vi "HOST_856.vi"() -> ()   [LabVIEW 2018]
uses:
  <vilib>/userdefined/High Color/nirio_resource_hc.ctl
  <instrlib>/niDCPower/nidcpower.llb/niDCPower Measurement Type.ctl
  <vilib>/FPGAPlugInAG/PXI-7953R/niLvFpga_Open_PXI-7953R.vi
  <vilib>/rvi/interface/common/dynamic/niFpgaDynamicAddResources.vi
  <vilib>/FPGAPlugInAG/Dynamic/niLvFpga_Reset_Dynamic.vi
  <vilib>/FPGAPlugInAG/Dynamic/niLvFpga_Run_Dynamic.vi
  <vilib>/Utility/error.llb/Error Cluster From Error Code.vi
  <vilib>/rvi/errors/niLvFpgaAdjustHostInterfaceError.vi
  <vilib>/FPGAPlugInAG/Dynamic/niLvFpga_Close_Dynamic.vi
  <vilib>/rvi/interface/nirviOpenFPGA/nirviOpenFPGA.xnode
  FPGA Bitfiles/856_FPGATarget_TARGET856_N743GwyKryU.lvbitx
  <vilib>/rvi/interface/nirviMethod/nirviMethod.xnode
  <vilib>/rvi/interface/nirviReadWriteControl/nirviReadWriteControl.xnode
  <vilib>/rvi/interface/nirviCloseFPGA/nirviCloseFPGA.xnode
  NiFpgaLv.dll
  <vilib>/rvi/interface/Simulation/niFpgaSimulationCallBeginRW.vi
  <vilib>/Analysis/NI_AALPro.lvlib
  <vilib>/FPGAPlugInAG/Dynamic/niLvFpga_ReadFifo_Dynamic.vi
  <vilib>/rvi/errors/niLvFpgaMergeErrorWithErrorCode.vi
panel:
  in  "Включаем автоматом?":bool
  out "2V":i32
  out "PH":i32
  out "RD":i32
  out "1V":i32
  out "-15":i32
  out "STAB":i32
  out "ADC":i32
  out "PS":i32
  out "DD":i32
  in  "НЕПРЕРЫВНО":bool
  in  "Частота?":enum16{"MIN", "MAX"}(ring)
  out "FRAME_OK":bool
  in  "Frames":path=path "C:/VPL/LabView_PRJ/DOZOR/856/FRAMES"
  in  "ПРИМЕЧАНИЕ":string
  in  "Запись Кадра":bool
  out "Image":T1(plugin-control)
  out "OUT":cluster{u16, u16, u16, u16}[][](array[cluster])
  out "FRAME":u16[][](array[numeric])
  out "Среднее":dbl
  in  "ISO":dbl=1.0
  out "СКО":dbl
  out "БД":i32
  in  "Усреднение":i32=2
  in  "Какая фотка?":string="1"
  out "Фотонная калибровка":cluster{dbl[], dbl[]}(graph)={[2945.34925, 4162.883, 5407.114, 6646.145, 7867.278, 9112.486, 10343.8485, 11629.84075, 12845.8065, 14105.4315, 15360.77375, 16587.11725, 17848.9395, 19098.027, 20350.598, 21566.6655, 22775.31325, 24040.47325, 25248.73825, 26509.4255, 27746.5745, 28973.666, 30216.06275, 31422.62225, 32653.4605, 33877.69175, 35109.20175, 36357.606, 37567.2215, 38767.47625, 39966.91875, 41163.4865, 42387.08325, 43594.03975, 44808.45875, 45970.48675, 46992.77825, 47671.652, 47865.0265, 47721.78775], [754.7077538726073, 1294.11479262345, 893.7580964968845, 980.3232389360018, 850.0287895485105, 1065.2375920249935, 1169.789721684937, 1100.165165964065, 1157.3372063515674, 1007.1309132404187, 1162.2567557572454, 1457.9632114764704, 1235.5849362859356, 1356.272022665283, 1233.965587313386, 1352.3965001901172, 1891.8062110466317, 1582.0298087255514, 1624.0064309213171, 1513.4693861032604, 1646.7886382482766, 1815.5518856486406, 2715.7512741820756, 2363.008614392699, 2216.4912798029472, 2054.855897832658, 1991.5005921076636, 2056.3553886491773, 2018.0820574154084, 2317.7418848882035, 2312.454466035146, 2381.6246235017934, 2156.6081452826106, 2313.878534130175, 2194.9621434641085, 2197.1906134834308, 3715.350346195178, 3050.689760121681, 6316.385477342978, 6689.87150748068]}
  out "Ке":dbl
  out "Светосигнальная":cluster{u8, "ДИСКРЕТ, мс":u8, dbl[]}(graph)={1, "ДИСКРЕТ, мс"=6, [2945.34925, 4162.883, 5407.114, 6646.145, 7867.278, 9112.486, 10343.8485, 11629.84075, 12845.8065, 14105.4315, 15360.77375, 16587.11725, 17848.9395, 19098.027, 20350.598, 21566.6655, 22775.31325, 24040.47325, 25248.73825, 26509.4255, 27746.5745, 28973.666, 30216.06275, 31422.62225, 32653.4605, 33877.69175, 35109.20175, 36357.606, 37567.2215, 38767.47625, 39966.91875, 41163.4865, 42387.08325, 43594.03975, 44808.45875, 45970.48675, 46992.77825, 47671.652, 47865.0265, 47721.78775]}
  out "Коэффициент наклона":dbl=207.02341506892228
  out "Ssat, АЦП":dbl
  out "Usat, В":dbl
  out "СКО выхода от выхода":cluster{dbl[], dbl[]}(graph)={[2945.34925, 4162.883, 5407.114, 6646.145, 7867.278, 9112.486, 10343.8485, 11629.84075, 12845.8065, 14105.4315, 15360.77375, 16587.11725, 17848.9395, 19098.027, 20350.598, 21566.6655, 22775.31325, 24040.47325, 25248.73825, 26509.4255, 27746.5745, 28973.666, 30216.06275, 31422.62225, 32653.4605, 33877.69175, 35109.20175, 36357.606, 37567.2215, 38767.47625, 39966.91875, 41163.4865, 42387.08325, 43594.03975, 44808.45875, 45970.48675, 46992.77825, 47671.652, 47865.0265, 47721.78775], [27.56116381795225, 39.4680052194179, 40.61277628714881, 48.477521595065056, 55.182654065838534, 67.51923353941456, 80.54674293694316, 88.70693386652474, 100.42434198938025, 112.23595038021465, 121.90756785368164, 135.55632205009846, 146.1681098589908, 159.01610695461008, 168.6889274367171, 181.34877002891415, 194.2995537044542, 205.61065872116154, 218.75093055744918, 230.2984198811404, 242.14403406030874, 255.5250241052722, 276.43391011958, 276.89883684118286, 291.2733485851393, 302.2832268581072, 315.62427374926335, 328.22661952376734, 338.672418007431, 352.34511163594993, 365.25131673273967, 377.41954602802423, 390.1457799845464, 400.77045170396485, 411.75904694827284, 399.1861749481692, 316.8742762670236, 156.11020272871326, 93.14512090147284, 141.78671742797337]}
  out "Эфф. по гор.":dbl
  out "Эфф. по верт.":dbl
  in  "ДИСКРЕТ, мс":u8=6
  in  "Кол-во итераций":i32=40
  in  "Расчет":bool
  in  "10":u8=20
  in  "PH11_1":u8=3
  in  "PH11_2":u8=13
  in  "PH21_1":u8=3
  in  "PH21_2":u8=13
  in  "RG_1":u8=3
  in  "PS4_2":u16=1371
  in  "PS4_1":u16=277
  in  "PS2_2":u16=1151
  in  "PS2_1":u16=496
  in  "2017":u16=2017
  in  "Какой канал?":enum16{"OUT1", "OUT2", "OUT3"}(ring)
  in  "文韧 世男!":bool
  in  "Линейки":bool
  in  "Сколько строк?":i32=110
  in  "Строка триггер":u16=50
  in  "PS1_2":u16=1809
  in  "PS1_1":u16=715
  in  "PS3_1":u16=934
  in  "PS3_2":u16=1589
  in  "CDS1_2":u8=13
  in  "CDS1_1":u8=5
  in  "CDS2_2":u8=16
  in  "CDS2_1":u8=2
  in  "ADC_2":u8=18
  in  "ADC_1":u8=7
  in  "RG_2":u8=5
  in  "HOR":u16=880
  in  "LOW":u8=7
  in  "HIGH":u8=18
  in  "Между кадрами, мс":u8=1
  in  "Прошить АЦП":bool
  out "АЦП прошит!":bool
  in  "Усиление (до 6)_OUT3":u8=1
  in  "Усиление (до 6)_OUT1":u8=1
  in  "Усиление (до 6)_OUT2":u8=1
  in  "Смещение, до 300_OUT1":dbl
  in  "+/- OUT1":enum16{"-", "+"}(ring)=enum."+"
  in  "Смещение, до 300_OUT3":dbl
  in  "+/- OUT3":enum16{"-", "+"}(ring)=enum."+"
  in  "Смещение, до 300_OUT2":dbl
  in  "+/- OUT2":enum16{"-", "+"}(ring)=enum."+"
  in  "2/4 V":enum16{"2V", "4V"}(ring)=enum."4V"
  in  "3CH/1CH":enum16{"3CH", "1CH"}(ring)=enum."1CH"
  out "Configuration":bool[](array[boolean])=[FALSE, FALSE, FALSE, TRUE, TRUE, FALSE, TRUE, TRUE, FALSE]
  out "ADC":bool
  out "STAB":bool
  in  "0,005":dbl=0.005 format="%#_13g"
  out "-15":bool
  out "1V":bool
  out "RD":bool
  out "PH":bool
  out "2V":bool
  out "DD":bool
  out "PS":bool
  in  "ADC, V":dbl=6.0 caption="voltage level" format="%_6p"
  in  "RD, V":dbl=14.499999999999998 caption="voltage level" format="%_6p"
  in  "PH_LOW, V":dbl=-4.000000000000002 caption="voltage level" format="%_6p"
  in  "DD, V":dbl=18.500000000000007 caption="voltage level" format="%_6p"
  in  "ADC_curlim":dbl=0.2 caption="current limit" format="%_6p"
  in  "STAB_curlim":dbl=0.2 caption="current limit" format="%_6p"
  in  "RD_curlim":dbl=0.1 caption="current limit" format="%_6p"
  in  "PH_LOW_curlim":dbl=0.1 caption="current limit" format="%_6p"
  in  "2V_curlim":dbl=0.1 caption="current limit" format="%_6p"
  in  "DD_curlim":dbl=0.1 caption="current limit" format="%_6p"
  out "ADC_cur":dbl caption="measurement" format="%_6g"
  out "STAB_cur":dbl caption="measurement" format="%_6g"
  out "RD_cur":dbl caption="measurement" format="%_6g"
  out "PH_LOW_cur":dbl caption="measurement" format="%_6g"
  out "2V_cur":dbl caption="measurement" format="%_6g"
  out "DD_cur":dbl caption="measurement" format="%_6g"
  in  "STAB, V":dbl=15.0 caption="voltage level" format="%_6p"
  in  "2V":dbl=2.0 caption="voltage level" format="%_6p"
  in  "1V":dbl=1.0 caption="voltage level" format="%_6p"
  in  "1V_curlim":dbl=0.1 caption="current limit" format="%_6p"
  out "1V_cur":dbl caption="measurement" format="%_6g"
  in  "-15_curlim":dbl=0.1 caption="current limit" format="%_6p"
  out "-15_cur":dbl caption="measurement" format="%_6g"
  in  "-15, V":dbl=-15.0 caption="voltage level" format="%_6p"
  in  "PS_LOW, V":dbl=-8.0 caption="voltage level" format="%_6p"
  in  "PS_LOW_curlim":dbl=0.1 caption="current limit" format="%_6p"
  out "PS_LOW_cur":dbl caption="measurement" format="%_6g"
  in  "Питание":bool
  in  "Стоп":bool
  in  "2":refnum<k15>="PXI1Slot4" caption="instrument handle"
  in  "0":refnum<k15>="PXI1Slot2" caption="instrument handle"
  in  "1":refnum<k15>="PXI1Slot3" caption="instrument handle"
  in  "resource name":T2="PXI1Slot5"
  in  "LOGS":path=path "C:/VPL/LabView_PRJ/DOZOR/856/LOGS"
  out "Номер образца":string="2"
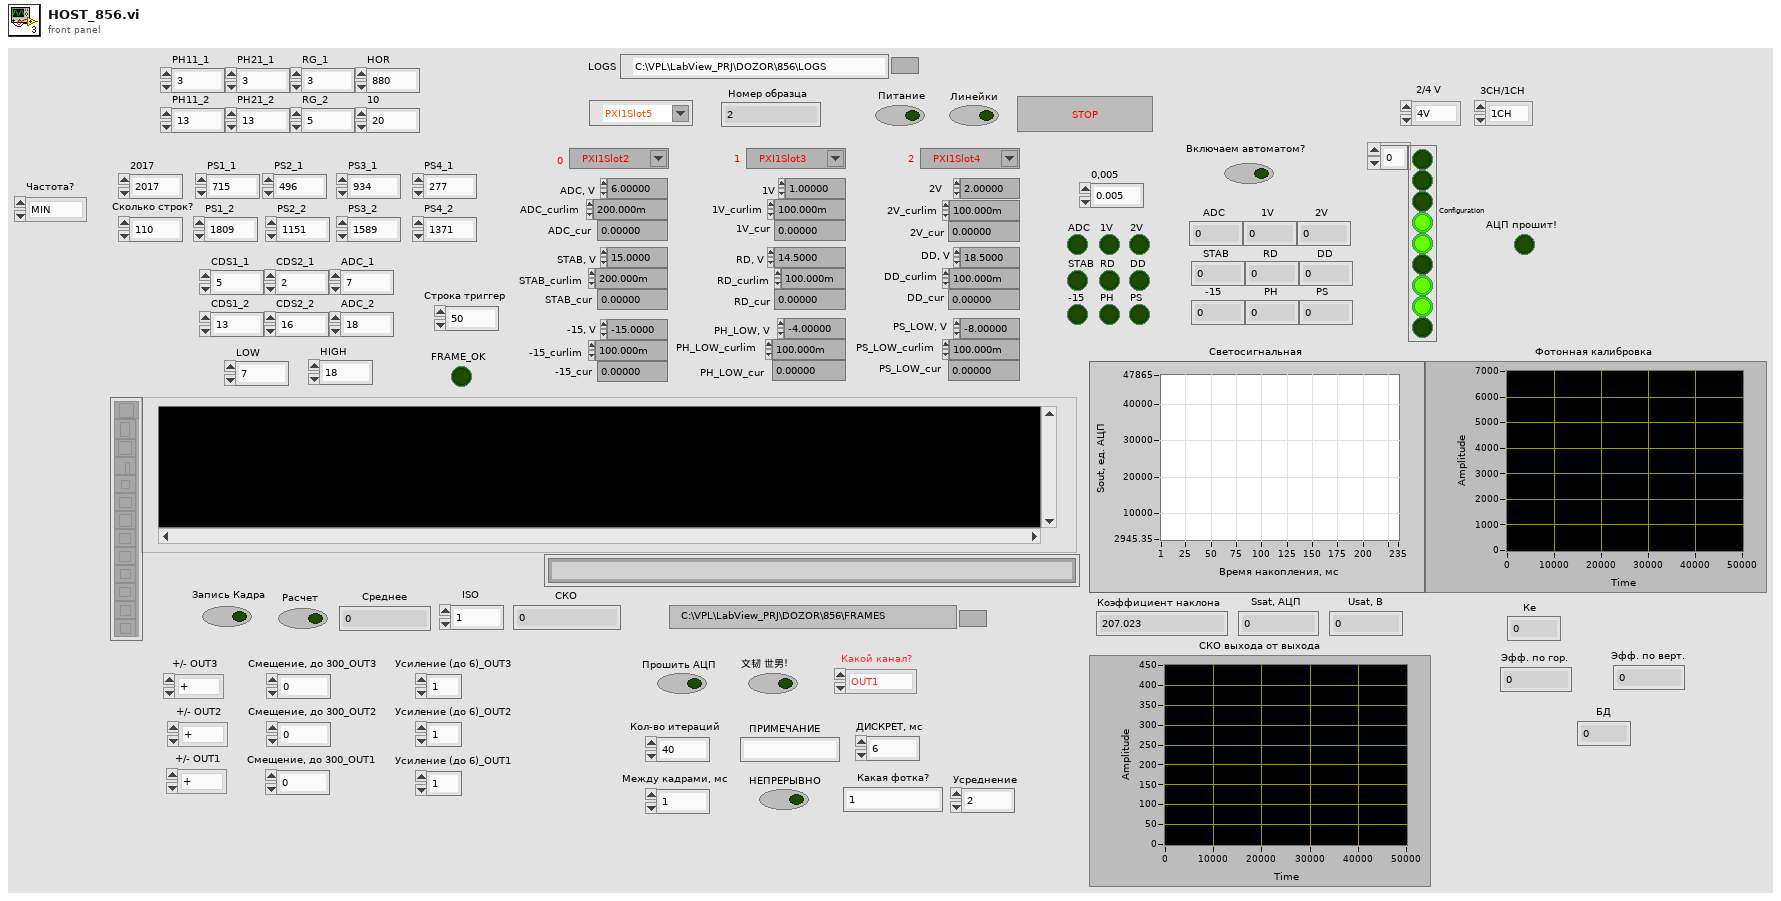
[diagram p1: front panel]
types:
  T1 = typedef "IMAQ Image.ctl" = refnum<image>
  T2 = typedef "nirio_resource_hc.ctl" = tag
  T3 = enum16{"open", "replace", "create", "open or create", "replace or create", "replace or create with confirmation"}
  T4 = typedef "niDCPower Measurement Type.ctl" = i32
  T5 = typedef "Image Type" = u32
  T6 = enum16{"Configuration", "MUX", "RED PGA", "GREEN PGA", "BLUE PGA", "RED OFF", "GREEN OFF", "BLUE OFF"}
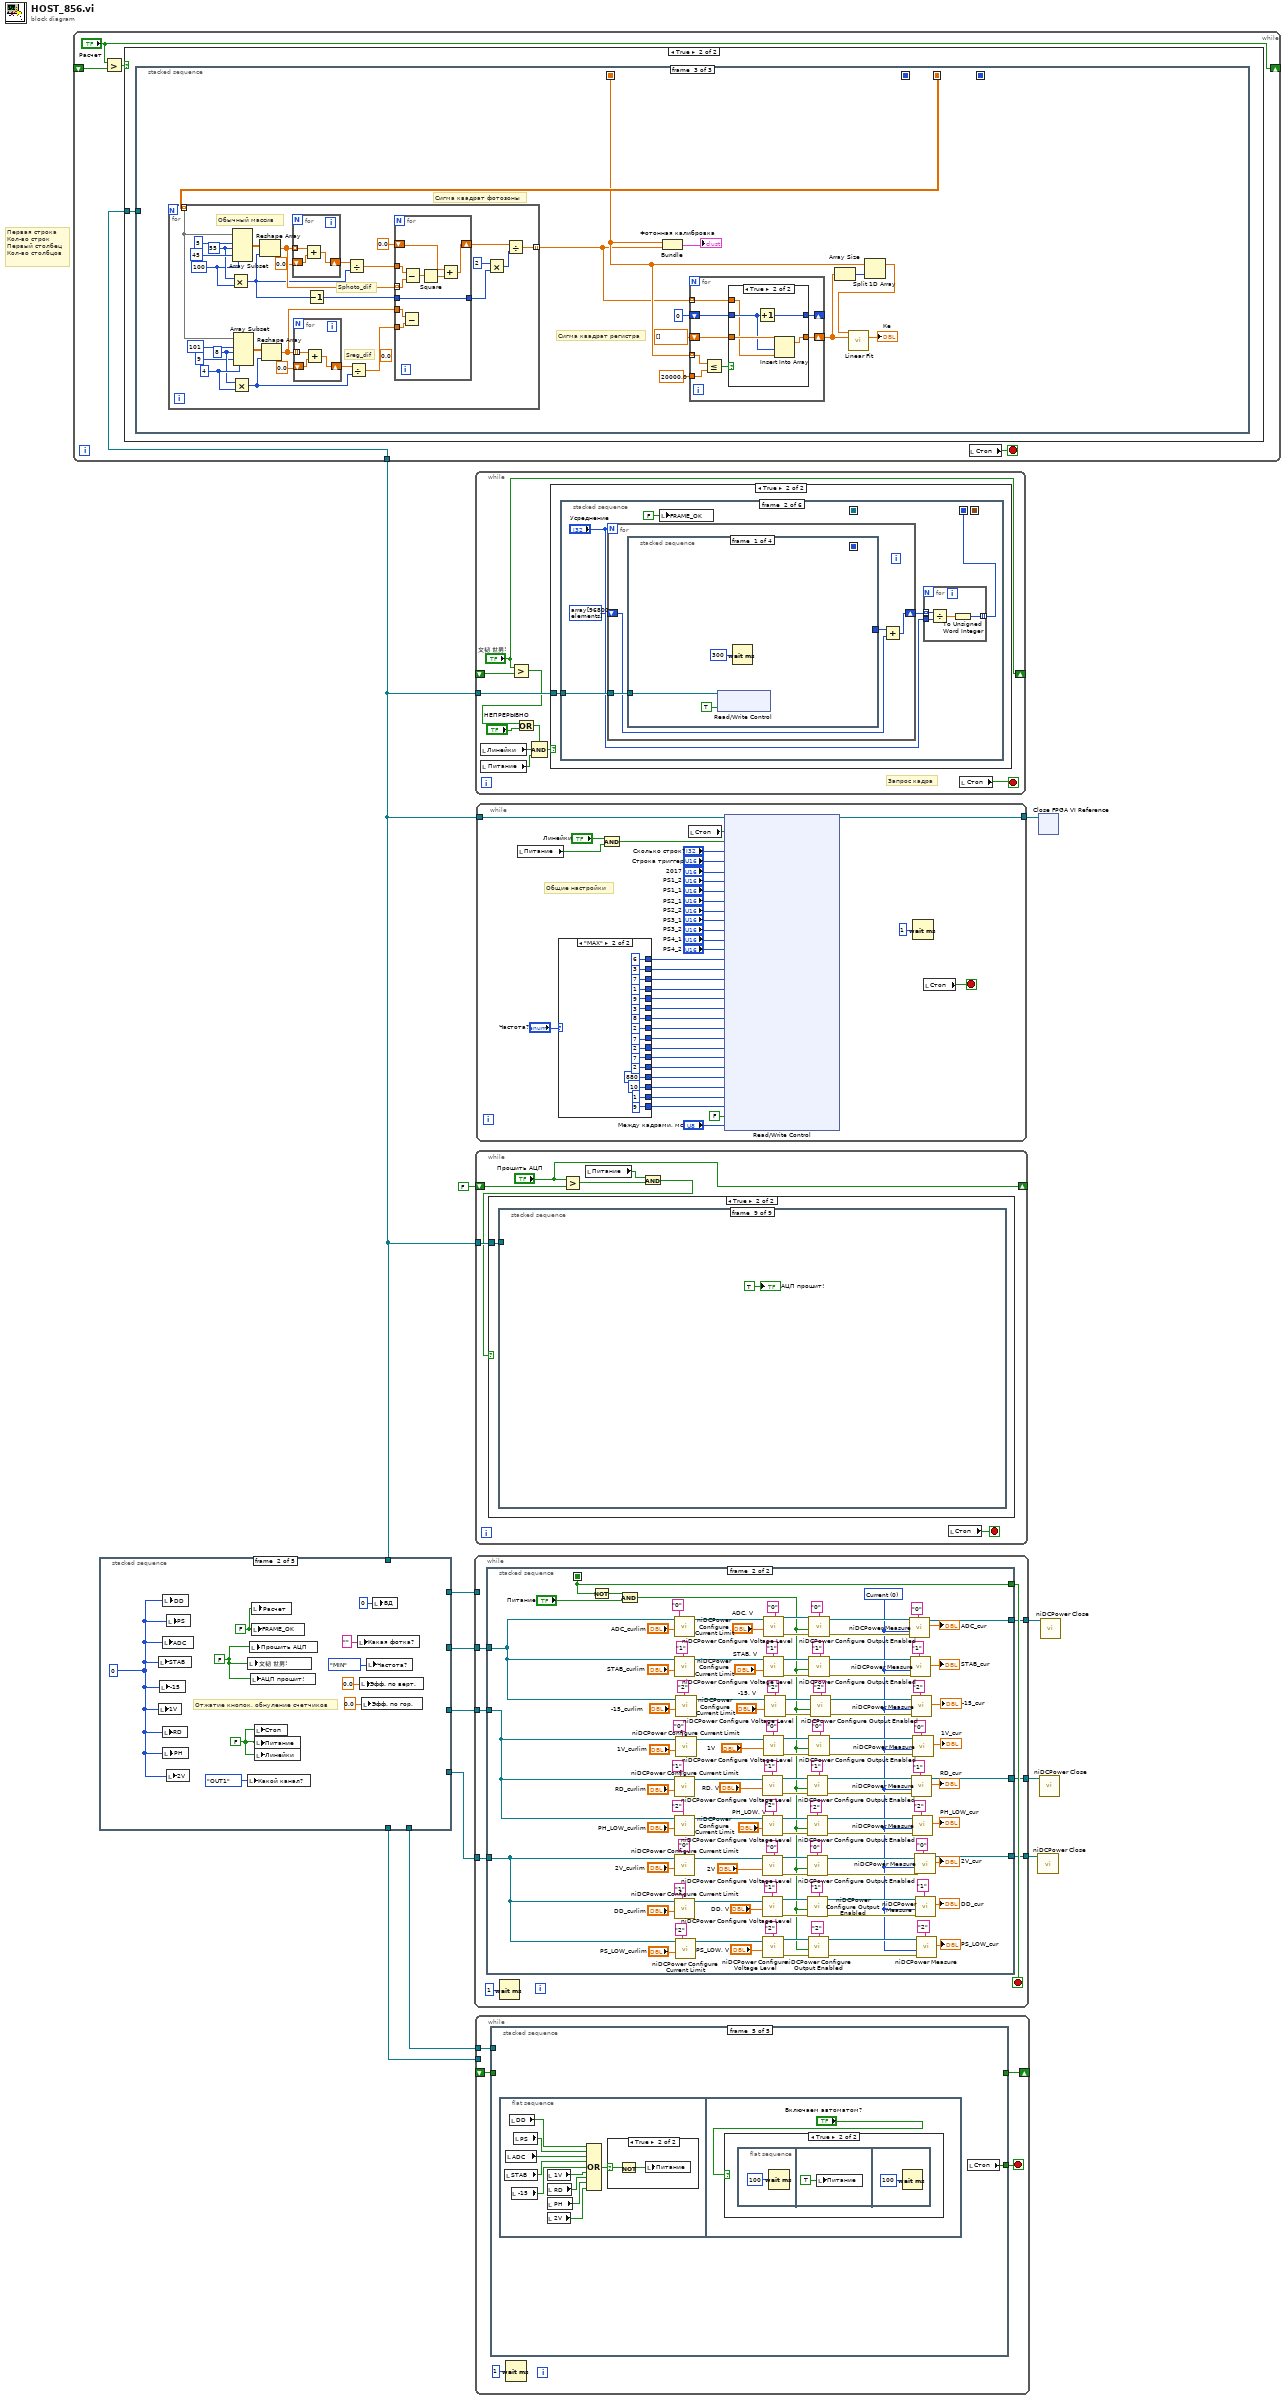
[diagram p0: block diagram]
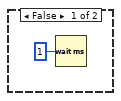
[diagram p2: hidden frame]
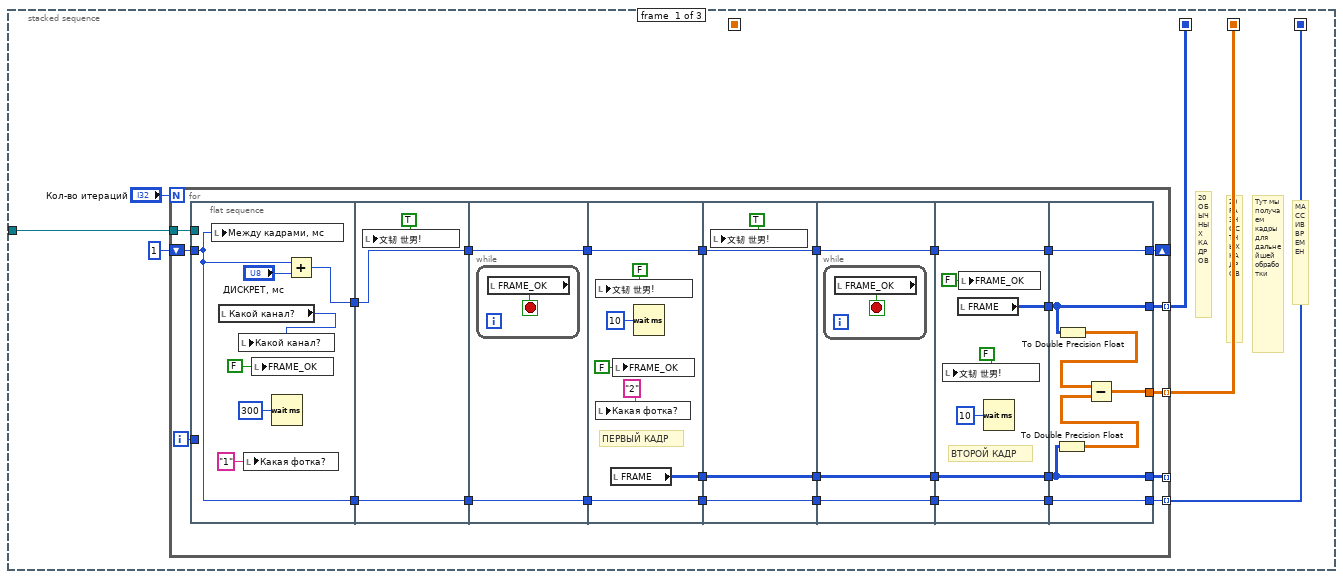
[diagram p3: hidden frame]
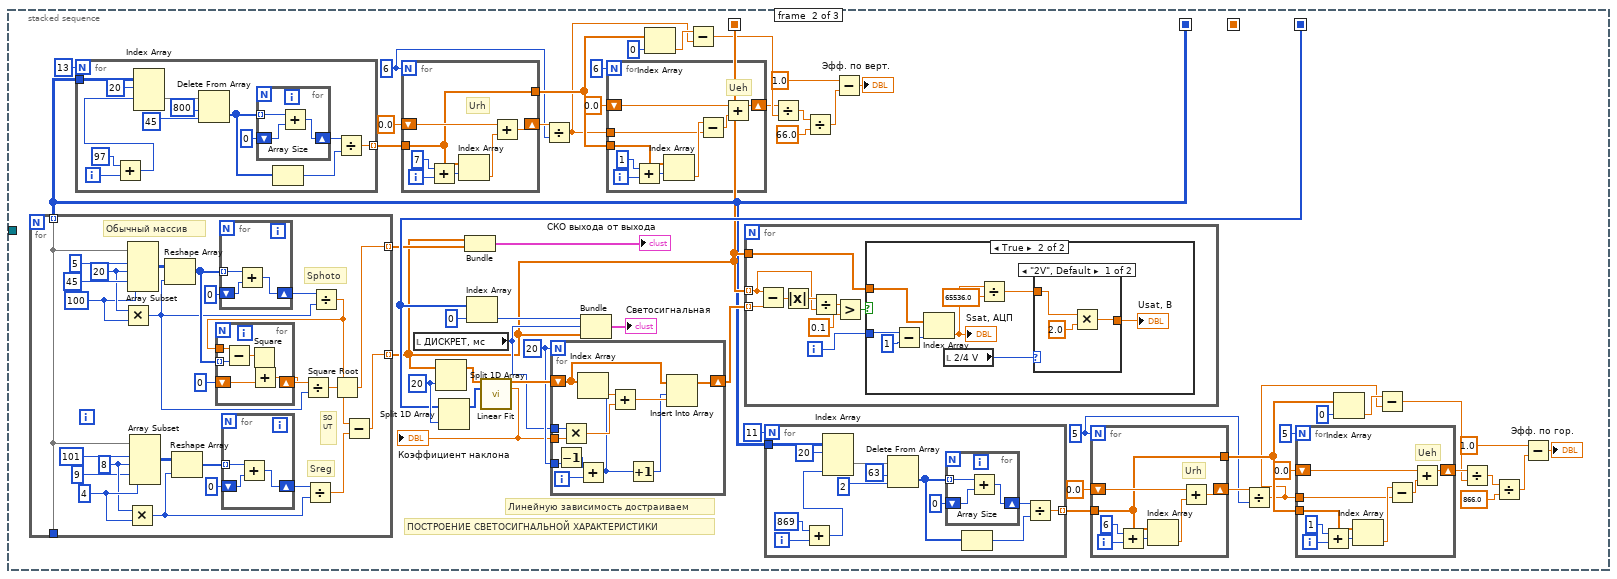
[diagram p4: hidden frame]
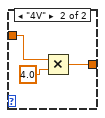
[diagram p6: hidden frame]
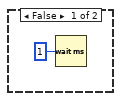
[diagram p8: hidden frame]
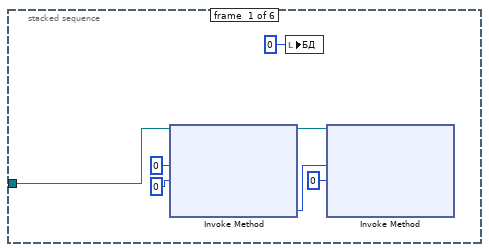
[diagram p9: hidden frame]
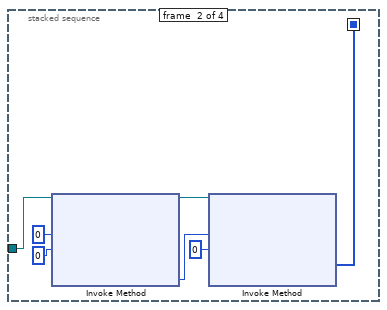
[diagram p10: hidden frame]
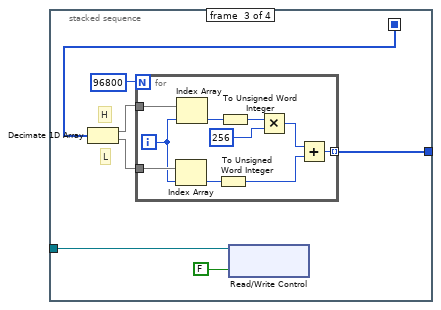
[diagram p11: hidden frame]
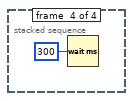
[diagram p12: hidden frame]
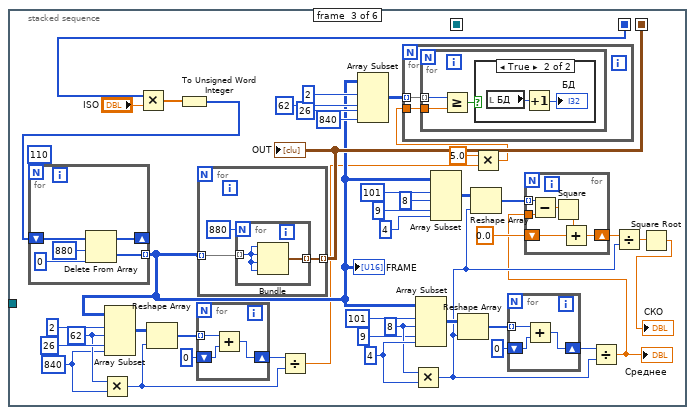
[diagram p13: hidden frame]
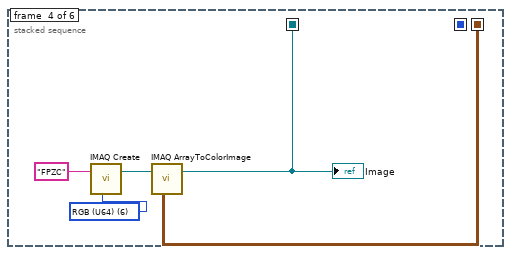
[diagram p15: hidden frame]
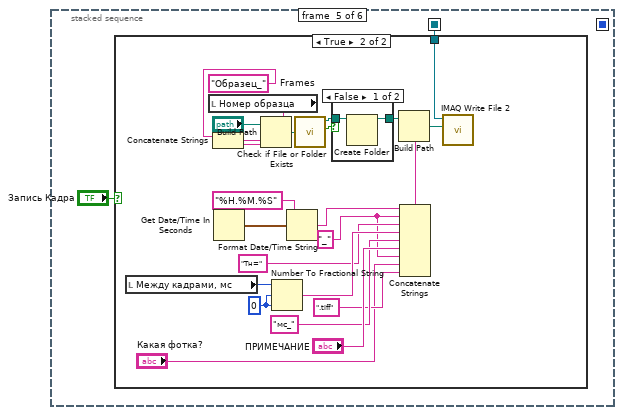
[diagram p16: hidden frame]
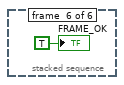
[diagram p19: hidden frame]
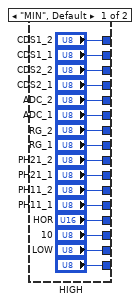
[diagram p20: hidden frame]
diagram:
  # "Первая строка\nКол-во строк\nПервый столбец\nКол-во столбцов"
  n1 = stacked-sequence {
    tunnel: [_ _ _ w61 _] -> w12
    tunnel: [_ _ _ _ w69] -> w9
    tunnel: [_ _ _ _ w68] -> w11
    tunnel: [_ _ _ _ w67] -> w10
    tunnel: [_ _ _ w61 _] -> w1
    tunnel: [_ _ _ w61 _] -> w5
    tunnel: [_ _ w24 _ _] -> w2
    frame #0 {
      n2 = call "Begin.vi"() -> ("Номер образца 2"=→"Номер образца":string)  [unwired: 11 in]
    }
    frame #1 {
      w14 = 0 ("DD")
      w21 = FALSE ("FRAME_OK")
      w22 = FALSE
      w23 = FALSE ("Стоп")
      # "Отжатие кнопок, обнуление счетчиков"
      n3 = local write "STAB"(w14) -> ()
      n4 = local write "1V"(w14) -> ()
      n5 = local write "-15"(w14) -> ()
      n6 = local write "ADC"(w14) -> ()
      n7 = local write "RD"(w14) -> ()
      n8 = local write "DD"(w14) -> ()
      n9 = local write "PH"(w14) -> ()
      n10 = local write "2V"(w14) -> ()
      n11 = local write "PS"(w14) -> ()
      n12 = local write "Какой канал?"(enum16{"OUT1", "OUT2", "OUT3"}."OUT1" ("Какой канал?")) -> ()
      n13 = local write "文韧 世男!"(w22) -> ()
      n14 = local write "Прошить АЦП"(w22) -> ()
      n15 = local write "АЦП прошит!"(w22) -> ()
      n16 = local write "FRAME_OK"(w21) -> ()
      n17 = local write "Расчет"(w21) -> ()
      n18 = local write "Стоп"(w23) -> ()
      n19 = local write "Питание"(w23) -> ()
      n20 = local write "Линейки"(w23) -> ()
      n21 = local write "Какая фотка?"("" ("Какая фотка?")) -> ()
      n22 = local write "Эфф. по верт."(0.0 ("Эфф. по верт.")) -> ()
      n23 = local write "Эфф. по гор."(0.0 ("Эфф. по гор.")) -> ()
      n24 = local write "Частота?"(enum16{"MIN", "MAX"}."MIN" ("Частота?")) -> ()
      n25 = local write "БД"(0 ("БД")) -> ()
    }
    frame #2 {
      w26 = "\t"
      n26 = local read "Номер образца"() -> (w53:string)
      n27 = Build Path(base path="LOGS", name or relative path=w53) -> (appended path=w50:path)
      n28 = Get Date/Time In Seconds() -> (seconds since 1Jan1904=w47:timestamp)
      n29 = call <vilib>:"Check if File or Folder Exists.vi"("path"=w50) -> ("file or folder exists?"=w51:bool, "dup path"=w52:path)  [unwired: 8 in, 1 out]
      n30 = Format Date/Time String(time format string (%c)="%d %H.%M.%S", seconds (now)=w47) -> (date/time string=w45:string)  [unwired: 1 in]
      n31 = case shown="False" w51 {
        tunnel: w52 -> [w59 w60]
        tunnel: [w58 w60] -> w42
        frame False {
          n32 = Create Folder(path (use dialog)=w59) -> (created path=w58:path)  [unwired: 2 in, 2 out]
        }
        frame True {
        }
      }
      n33 = Concatenate Strings(w45, ".xls" ("string")) -> (w44:string)
      n34 = Build Path(base path=w42, name or relative path=w44) -> (appended path=w46:path)
      n35 = Open/Create/Replace File(file path (use dialog)=w46, operation (0:open)=T3."open or create", access (0:read/write)=enum16{"read/write", "read-only", "write-only"}."read/write") -> (refnum out=w48:refnum<file>)  [unwired: 3 in, 2 out]
      n36 = case shown="True" TRUE {
        tunnel: w48 -> [w54 w57]
        tunnel: [w54 w55] -> w43
        frame False {
        }
        frame True {
          n37 = Set File Position(refnum=w57, from (0:start)=enum16{"start", "end", "current"}."end") -> (refnum out=w55:refnum<file>)  [unwired: 2 in, 1 out]
        }
      }
      n38 = Format Into String(initial string=w43, "Time" ("input 1"), w26, "ADC_cur", w26, "STAB_cur", w26, "-15_cur", w26, "1_cur", w26, "RD_cur", w26, "PH_LOW_cur", w26, "2V_cur", w26, "DD_cur", w26, "PS_LOW_cur", "\r\n") -> (resulting string=w24:refnum<file>)  [unwired: 2 in, 1 out]
    }
    frame #3 {
      n39 = xnode "Open FPGA VI Reference"("resource name"="resource name") -> ("FPGA VI Reference Out"=w62:refnum<k20>, "error out"=w64:errorcluster)  [unwired: 1 in]
      n40 = xnode "Invoke Method"("FPGA VI Reference In"=w62, "error in"=w64) -> ("FPGA VI Reference Out"=w65:refnum<k20>, "error out"=w63:errorcluster)
      n41 = xnode "Invoke Method"("FPGA VI Reference In"=w65, "error in"=w63) -> ("FPGA VI Reference Out"=w61:refnum<k20>)  [unwired: 1 in, 1 out]
    }
    frame #4 {
      n42 = call <instrlib>:"niDCPower Initialize.vi"("resource name"="2") -> ("error out"=w75:errorcluster, "instrument handle out"=w72:refnum<k15>)  [unwired: 3 in, 6 out]
      n43 = call <instrlib>:"niDCPower Initialize.vi"("resource name"="1") -> ("error out"=w73:errorcluster, "instrument handle out"=w70:refnum<k15>)  [unwired: 3 in, 6 out]
      n44 = call <instrlib>:"niDCPower Initialize.vi"("resource name"="0") -> ("error out"=w74:errorcluster, "instrument handle out"=w71:refnum<k15>)  [unwired: 3 in, 6 out]
      n45 = call <instrlib>:"niDCPower Configure Voltage Level.vi"("error in (no error)"=w75, "voltage level"=0.0, "channel name"="0,1,2", "instrument handle"=w72) -> ("instrument handle out"=w69:refnum<k15>)  [unwired: 6 in, 1 out]
      n46 = call <instrlib>:"niDCPower Configure Voltage Level.vi"("error in (no error)"=w73, "voltage level"=0.0, "channel name"="0,1,2", "instrument handle"=w70) -> ("instrument handle out"=w67:refnum<k15>)  [unwired: 6 in, 1 out]
      n47 = call <instrlib>:"niDCPower Configure Voltage Level.vi"("error in (no error)"=w74, "voltage level"=0.0, "channel name"="0,1,2", "instrument handle"=w71) -> ("instrument handle out"=w68:refnum<k15>)  [unwired: 6 in, 1 out]
    }
  }
  n48 = while {
    shift-right: ["Расчет"] -> _
    shift-left: _ -> [w87]
    tunnel: w1 -> [w85]
    stop <- w89 stop-if-true
    n49 = Greater?(x="Расчет", y=w87) -> (0:w88:bool)
    n50 = case shown="True" w88 {
      tunnel: w85 -> [_ w91]
      frame False {
        n51 = Wait (ms)(milliseconds to wait=u32 1) -> ()  [unwired: 1 out]
      }
      frame True {
        n52 = stacked-sequence {
          seq-local: [w92 _ _] -> [_ w167 _]
          seq-local: [w94 _ _] -> [_ _ w367]
          seq-local: [w93 _ _] -> [_ w209 _]
          seq-local: [_ w204 _] -> [_ _ w359]
          tunnel: w91 -> [w97 _ _]
          frame #0 {
            # "МАССИВ ВРЕМЕН"
            # "Тут мы получаем кадры\nдля дальнейшей обработки"
            # "20 РАЗНОСТНЫХ КАДРОВ"
            # "20 ОБЫЧНЫХ КАДРОВ"
            n53 = for {
              N: "Кол-во итераций" -> [_]
              tunnel: w97 -> [w124]
              shift-right: [w122] -> _
              shift-left: u8 1 -> [w123]
              tunnel: [w109] -> w92 mode=indexing
              tunnel: [w108] -> w94 mode=indexing
              tunnel: [w107] -> w93 mode=indexing
              tunnel: [w98] -> _ mode=indexing
              i -> [w99]
              n54 = flat-sequence {
                tunnel: w124 -> [_]
                tunnel: w123 -> [w127]
                tunnel: [w130] -> w119
                tunnel: [w127] -> w100
                tunnel: w99 -> [_]
                tunnel: [w134] -> w121
                tunnel: w119 -> [w134]
                tunnel: [w132] -> w101
                tunnel: w100 -> [w132]
                tunnel: w121 -> [w136]
                tunnel: [w136] -> w120
                tunnel: [w135] -> w102
                tunnel: w101 -> [w135]
                tunnel: w120 -> [w144]
                tunnel: [w144] -> w118
                tunnel: [w141] -> w110
                tunnel: [w139] -> w103
                tunnel: w102 -> [w139]
                tunnel: w118 -> [w148]
                tunnel: [w148] -> w117
                tunnel: [w146] -> w111
                tunnel: w110 -> [w146]
                tunnel: [w145] -> w104
                tunnel: w103 -> [w145]
                tunnel: w117 -> [w151]
                tunnel: [w151] -> w116
                tunnel: [w150] -> w112
                tunnel: w111 -> [w150]
                tunnel: [w149] -> w105
                tunnel: w104 -> [w149]
                tunnel: w116 -> [w159]
                tunnel: [w159] -> w115
                tunnel: [w158] -> w114
                tunnel: [w157] -> w113
                tunnel: w112 -> [w157]
                tunnel: [w153] -> w106
                tunnel: w105 -> [w153]
                tunnel: [w166] -> w122
                tunnel: w115 -> [w166]
                tunnel: w114 -> [w164]
                tunnel: w113 -> [w160]
                tunnel: [w163] -> w108
                tunnel: [w164] -> w109
                tunnel: [w165] -> w107
                tunnel: w106 -> [w165]
                tunnel: [w160] -> w98
                frame #0 {
                  n55 = local write "Между кадрами, мс"(w127) -> ()
                  n56 = local read "Какой канал?"() -> (w126:enum16{"OUT1", "OUT2", "OUT3"})
                  n57 = local write "Какой канал?"(w126) -> ()
                  n58 = local write "Какая фотка?"("1" ("Какая фотка?")) -> ()
                  n59 = local write "FRAME_OK"(FALSE ("FRAME_OK")) -> ()
                  n60 = Wait (ms)(milliseconds to wait=u32 300) -> ()  [unwired: 1 out]
                  n61 = Add(x=w127, y="ДИСКРЕТ, мс") -> (x+y=w130:u8)
                }
                frame #1 {
                  n62 = local write "文韧 世男!"(TRUE ("文韧 世男!")) -> ()
                }
                frame #2 {
                  n63 = while {
                    stop <- w137 stop-if-true
                    n64 = local read "FRAME_OK"() -> (w137:bool)
                  }
                }
                frame #3 {
                  # "ПЕРВЫЙ КАДР"
                  n65 = local write "文韧 世男!"(FALSE ("文韧 世男!")) -> ()
                  n66 = local write "Какая фотка?"("2" ("Какая фотка?")) -> ()
                  n67 = local read "FRAME"() -> (w141:u16[][])
                  n68 = local write "FRAME_OK"(FALSE ("FRAME_OK")) -> ()
                  n69 = Wait (ms)(milliseconds to wait=u32 10) -> ()  [unwired: 1 out]
                }
                frame #4 {
                  n70 = local write "文韧 世男!"(TRUE ("文韧 世男!")) -> ()
                }
                frame #5 {
                  n71 = while {
                    stop <- w152 stop-if-true
                    n72 = local read "FRAME_OK"() -> (w152:bool)
                  }
                }
                frame #6 {
                  # "ВТОРОЙ КАДР"
                  n73 = local write "文韧 世男!"(FALSE ("文韧 世男!")) -> ()
                  n74 = local read "FRAME"() -> (w158:u16[][])
                  n75 = local write "FRAME_OK"(FALSE ("FRAME_OK")) -> ()
                  n76 = Wait (ms)(milliseconds to wait=u32 10) -> ()  [unwired: 1 out]
                }
                frame #7 {
                  n77 = To Double Precision Float(number=w160) -> (double precision float=w161:dbl[][])
                  n78 = To Double Precision Float(number=w164) -> (double precision float=w162:dbl[][])
                  n79 = Subtract(x=w162, y=w161) -> (x-y=w163:dbl[][])
                }
              }
            }
          }
          frame #1 {
            w169 = 6
            w170 = 5
            w212 = 20
            w217 = 20 ("index")
            # "ПОСТРОЕНИЕ СВЕТОСИГНАЛЬНОЙ ХАРАКТЕРИСТИКИ"
            # "Линейную зависимость достраиваем"
            n80 = for {
              tunnel: w167 -> [w319] mode=indexing
              tunnel: [w321] -> w204 mode=indexing
              tunnel: [w325] -> w206 mode=indexing
              tunnel: [w319] -> _
              w332 = 4 ("length")
              w331 = 8 ("length")
              w341 = 100 ("length")
              w342 = 20 ("length")
              # "SOUT"
              # "Sreg"
              # "Sphoto"
              # "Обычный массив"
              n81 = Multiply(x=w342, y=w341) -> (x*y=w323:i32)
              n82 = Multiply(x=w331, y=w332) -> (x*y=w337:i32)
              n83 = Array Subset(array=w319, index (row)=5 ("index"), length (row)=w342, index (col)=45 ("index"), length (col)=w341) -> (w340:u16[][])
              n84 = Array Subset(array=w319, index (row)=101 ("index"), length (row)=w331, index (col)=9 ("index"), length (col)=w332) -> (w333:u16[][])
              n85 = Reshape Array(w340, w323) -> (w327:u16[])
              n86 = Reshape Array(w333, w337) -> (w334:u16[])
              n87 = for {
                tunnel: w327 -> [w356] mode=indexing
                shift-right: [w354] -> w338
                shift-left: u64 0 -> [w355]
                n88 = Add(x=w356, y=w355) -> (x+y=w354:u64)
              }
              n89 = for {
                tunnel: w334 -> [w353] mode=indexing
                shift-right: [w351] -> w336
                shift-left: u64 0 -> [w352]
                n90 = Add(x=w353, y=w352) -> (x+y=w351:u64)
              }
              n91 = Divide(x=w336, y=w337) -> (x/y=w328:dbl)
              n92 = Divide(x=w338, y=w323) -> (x/y=w320:dbl)
              n93 = for {
                tunnel: w327 -> [w350] mode=indexing
                shift-right: [w349] -> w324
                shift-left: u64 0 -> [w346]
                tunnel: w320 -> [w345]
                n94 = Subtract(x=w345, y=w350) -> (x-y=w348:dbl)
                n95 = Square(x=w348) -> (x^2=w347:dbl)
                n96 = Add(x=w347, y=w346) -> (x+y=w349:dbl)
              }
              n97 = Divide(x=w324, y=w323) -> (x/y=w322:dbl)
              n98 = Square Root(x=w322) -> (sqrt(x)=w325:dbl)
              n99 = Subtract(x=w320, y=w328) -> (x-y=w321:dbl)
            }
            n100 = for {
              N: 13 -> [_]
              tunnel: w167 -> [w247]
              tunnel: [w236] -> w176 mode=indexing
              i -> [w238]
              n101 = Add(x=97, y=w238) -> (x+y=w235:i32)
              n102 = Index Array(array=w247, index (dim 0)=20 ("disabled index (page)"), index (dim 1)=w235) -> (element=w245:u16[])  [unwired: 1 in]
              n103 = Delete From Array(array=w245, length=800, index=45) -> (deleted portion=w240:u16[])  [unwired: 1 out]
              n104 = for {
                tunnel: w240 -> [w250] mode=indexing
                shift-right: [w248] -> w241
                shift-left: 0 -> [w249]
                n105 = Add(x=w250, y=w249) -> (x+y=w248:i32)
              }
              n106 = Array Size(array=w240) -> (size(s)=w239:i32)
              n107 = Divide(x=w241, y=w239) -> (x/y=w236:dbl)
            }
            n108 = for {
              N: w169 -> [_]
              tunnel: w176 -> [w228]
              shift-right: [w229] -> w172
              shift-left: 0.0 -> [w231]
              tunnel: [w228] -> w181
              i -> [w234]
              # "Urh"
              n109 = Add(x=7, y=w234) -> (x+y=w232:i32)
              n110 = Index Array(array=w228, index=w232) -> (element=w230:dbl)
              n111 = Add(x=w231, y=w230) -> (x+y=w229:dbl)
            }
            n112 = local read "ДИСКРЕТ, мс"() -> (w210:u8)
            n113 = Split 1D Array(array=w204, index=w217) -> (first subarray=w216:dbl[])  [unwired: 1 out]
            n114 = Split 1D Array(array=w209, index=w217) -> (first subarray=w215:u8[])  [unwired: 1 out]
            n115 = Bundle(w204, w206) -> (→"СКО выхода от выхода":cluster{dbl[], dbl[]})  [unwired: 1 in]
            n116 = Index Array(array=w209, index=0) -> (element=w214:u8)
            n117 = call <vilib>:"Linear Fit.vi"("Y"=w216, "X"=w215) -> ("Best Linear Fit"=w213:dbl[], "slope"=w211:dbl)  [unwired: 9 in, 3 out]
            "Коэффициент наклона" <- w211
            n118 = Divide(x=w172, y=w169) -> (x/y=w168:dbl)
            n119 = for {
              N: w212 -> [_]
              tunnel: w212 -> [w308]
              shift-right: [w316] -> w208
              shift-left: w213 -> [w309]
              tunnel: w211 -> [w315]
              tunnel: w210 -> [w314]
              i -> [w318]
              n120 = Decrement(x=w308) -> (x-1=w307:i32)
              n121 = Multiply(x=w314, y=w315) -> (x*y=w313:dbl)
              n122 = Add(x=w307, y=w318) -> (x+y=w311:i32)
              n123 = Index Array(array=w309, index=w311) -> (element=w317:dbl)
              n124 = Add(x=w317, y=w313) -> (x+y=w312:dbl)
              n125 = Increment(x=w311) -> (x+1=w310:i32)
              n126 = Insert Into Array(array=w309, index=w310, new element=w312) -> (w316:dbl[])
            }
            n127 = Bundle(w214, "ДИСКРЕТ, мс"=w210, w204) -> (→"Светосигнальная":cluster{u8, "ДИСКРЕТ, мс":u8, dbl[]})  [unwired: 1 in]
            n128 = for {
              N: 6 -> [_]
              tunnel: w181 -> [w224]
              shift-right: [w219] -> w179
              shift-left: 0.0 -> [w220]
              tunnel: w168 -> [w222]
              i -> [w227]
              # "Ueh"
              n129 = Add(x=1, y=w227) -> (x+y=w225:i32)
              n130 = Index Array(array=w224, index=w225) -> (element=w223:dbl)
              n131 = Subtract(x=w223, y=w222) -> (x-y=w221:dbl)
              n132 = Add(x=w220, y=w221) -> (x+y=w219:dbl)
            }
            n133 = Index Array(array=w181, index=0) -> (element=w182:dbl)
            n134 = Subtract(x=w182, y=w168) -> (x-y=w183:dbl)
            n135 = for {
              tunnel: w204 -> [w283] mode=indexing
              tunnel: w208 -> [w291] mode=indexing
              tunnel: w204 -> [w286]
              i -> [w287]
              n136 = Subtract(x=w283, y=w291) -> (x-y=w284:dbl)
              n137 = Absolute Value(x=w284) -> (abs(x)=w285:dbl)
              n138 = Divide(x=w285, y=w283) -> (x/y=w290:dbl)
              n139 = Greater?(x=w290, y=0.1) -> (0:w288:bool)
              n140 = case shown="True" w288 {
                tunnel: w287 -> [_ w294]
                tunnel: w286 -> [_ w300]
                frame False {
                }
                frame True {
                  n141 = Subtract(x=w294, y=1) -> (x-y=w295:i32)
                  n142 = Index Array(array=w300, index=w295) -> (element=w298:dbl)
                  "Ssat, АЦП" <- w298
                  n143 = local read "2/4 V"() -> (w299:enum16{"2V", "4V"})
                  n144 = Divide(x=w298, y=65536.0) -> (x/y=w296:dbl)
                  n145 = case shown="\"2V\", Default" w299 {
                    tunnel: w296 -> [w302 w306]
                    tunnel: [w301 w304] -> w292
                    frame "2V", Default {
                      n146 = Multiply(x=w302, y=2.0) -> (x*y=w301:dbl)
                    }
                    frame "4V" {
                      n147 = Multiply(x=w306, y=4.0) -> (x*y=w304:dbl)
                    }
                  }
                  "Usat, В" <- w292
                }
              }
            }
            n148 = for {
              N: 11 -> [_]
              tunnel: w167 -> [w279]
              tunnel: [w267] -> w202 mode=indexing
              i -> [w270]
              n149 = Add(x=869, y=w270) -> (x+y=w268:i32)
              n150 = Index Array(array=w279, index (dim 0)=20 ("disabled index (page)"), index (dim 2)=w268) -> (element=w277:u16[])  [unwired: 1 in]
              n151 = Delete From Array(array=w277, length=63, index=2) -> (deleted portion=w272:u16[])  [unwired: 1 out]
              n152 = for {
                tunnel: w272 -> [w282] mode=indexing
                shift-right: [w280] -> w273
                shift-left: 0 -> [w281]
                n153 = Add(x=w282, y=w281) -> (x+y=w280:i32)
              }
              n154 = Array Size(array=w272) -> (size(s)=w271:i32)
              n155 = Divide(x=w273, y=w271) -> (x/y=w267:dbl)
            }
            n156 = Divide(x=w179, y=w183) -> (x/y=w185:dbl)
            n157 = Divide(x=w185, y=66.0) -> (x/y=w187:dbl)
            n158 = Subtract(x=1.0, y=w187) -> (x-y=→"Эфф. по верт.":dbl)
            n159 = for {
              N: w170 -> [_]
              tunnel: w202 -> [w260]
              shift-right: [w261] -> w195
              shift-left: 0.0 -> [w263]
              tunnel: [w260] -> w197
              i -> [w266]
              # "Urh"
              n160 = Add(x=6, y=w266) -> (x+y=w264:i32)
              n161 = Index Array(array=w260, index=w264) -> (element=w262:dbl)
              n162 = Add(x=w263, y=w262) -> (x+y=w261:dbl)
            }
            n163 = Divide(x=w195, y=w170) -> (x/y=w171:dbl)
            n164 = for {
              N: 5 -> [_]
              tunnel: w197 -> [w256]
              shift-right: [w251] -> w199
              shift-left: 0.0 -> [w252]
              tunnel: w171 -> [w254]
              i -> [w259]
              # "Ueh"
              n165 = Add(x=1, y=w259) -> (x+y=w257:i32)
              n166 = Index Array(array=w256, index=w257) -> (element=w255:dbl)
              n167 = Subtract(x=w255, y=w254) -> (x-y=w253:dbl)
              n168 = Add(x=w252, y=w253) -> (x+y=w251:dbl)
            }
            n169 = Index Array(array=w197, index=0) -> (element=w196:dbl)
            n170 = Subtract(x=w196, y=w171) -> (x-y=w194:dbl)
            n171 = Divide(x=w199, y=w194) -> (x/y=w192:dbl)
            n172 = Divide(x=w192, y=866.0) -> (x/y=w190:dbl)
            n173 = Subtract(x=1.0, y=w190) -> (x-y=→"Эфф. по гор.":dbl)
          }
          frame #2 {
            # "Сигма квадрат регистра"
            # "Сигма квадрат фотозоны"
            n174 = for {
              tunnel: w367 -> [w398] mode=indexing
              tunnel: [w383] -> w358 mode=indexing
              (unwired) 0.0
              w402 = 4 ("length")
              w401 = 8 ("length")
              w407 = 100 ("length")
              w408 = 55 ("length")
              # "Sreg_dif"
              # "Sphoto_dif"
              # "Обычный массив"
              n175 = Multiply(x=w408, y=w407) -> (x*y=w393:i32)
              n176 = Multiply(x=w401, y=w402) -> (x*y=w391:i32)
              n177 = Array Subset(array=w398, index (row)=5 ("index"), length (row)=w408, index (col)=45 ("index"), length (col)=w407) -> (w406:dbl[][])
              n178 = Array Subset(array=w398, index (row)=101 ("index"), length (row)=w401, index (col)=9 ("index"), length (col)=w402) -> (w403:dbl[][])
              n179 = Reshape Array(w406, w393) -> (w396:dbl[])
              n180 = Reshape Array(w403, w391) -> (w395:dbl[])
              n181 = for {
                tunnel: w396 -> [w425] mode=indexing
                shift-right: [w423] -> w405
                shift-left: 0.0 -> [w424]
                n182 = Add(x=w425, y=w424) -> (x+y=w423:dbl)
              }
              n183 = for {
                tunnel: w395 -> [w422] mode=indexing
                shift-right: [w420] -> w404
                shift-left: 0.0 -> [w421]
                n184 = Add(x=w422, y=w421) -> (x+y=w420:dbl)
              }
              n185 = Decrement(x=w393) -> (x-1=w392:i32)
              n186 = Divide(x=w405, y=w393) -> (x/y=w387:dbl)
              n187 = Divide(x=w404, y=w391) -> (x/y=w397:dbl)
              n188 = for {
                tunnel: w387 -> [w417]
                tunnel: w397 -> [w418]
                tunnel: w396 -> [w416] mode=indexing
                tunnel: w395 -> [w419]
                shift-right: [w412] -> w394
                shift-left: 0.0 -> [w413]
                tunnel: [w411] -> w388
                tunnel: w392 -> [w411]
                n189 = Subtract(x=w419, y=w418) -> ()  [unwired: 1 out]
                n190 = Subtract(x=w417, y=w416) -> (x-y=w415:dbl)
                n191 = Square(x=w415) -> (x^2=w414:dbl)
                n192 = Add(x=w413, y=w414) -> (x+y=w412:dbl)
              }
              n193 = Multiply(x=2, y=w388) -> (x*y=w389:i32)
              n194 = Divide(x=w394, y=w389) -> (x/y=w383:dbl)
            }
            n195 = Bundle(w359, w358) -> (→"Фотонная калибровка":cluster{dbl[], dbl[]})  [unwired: 1 in]
            n196 = for {
              tunnel: w359 -> [w373] mode=indexing
              tunnel: 20000.0 -> [w375]
              shift-right: [w369] -> w364
              shift-left: dbl[] [] -> [w372]
              shift-right: [w370] -> _
              shift-left: 0 -> [w371]
              tunnel: w358 -> [w368] mode=indexing
              n197 = Less Or Equal?(x=w373, y=w375) -> (x <= y?=w374:bool)
              n198 = case shown="True" w374 {
                tunnel: w372 -> [w376 w382]
                tunnel: w371 -> [w377 w380]
                tunnel: [w377 w381] -> w370
                tunnel: [w376 w379] -> w369
                tunnel: w368 -> [_ w378]
                frame False {
                }
                frame True {
                  n199 = Increment(x=w380) -> (x+1=w381:i32)
                  n200 = Insert Into Array(array=w382, index=w380, new element=w378) -> (w379:dbl[])
                }
              }
            }
            n201 = Array Size(array=w364) -> (size(s)=w363:i32)
            n202 = Split 1D Array(array=w359, index=w363) -> (first subarray=w362:dbl[])  [unwired: 1 out]
            n203 = call <vilib>:"Linear Fit.vi"("Y"=w362, "X"=w364) -> ("slope"=→"Ке":dbl)  [unwired: 9 in, 4 out]
          }
        }
      }
    }
    n204 = local read "Стоп"() -> (w89:bool)
  }
  n205 = while {
    tunnel: w12 -> [_]
    tunnel: w11 -> [w432]
    tunnel: w10 -> [w431]
    tunnel: w9 -> [w430]
    tunnel: [w428] -> w8
    tunnel: [w427] -> w7
    tunnel: [w426] -> w6
    stop <- w429 stop-if-true
    n206 = stacked-sequence {
      seq-local: ["Стоп" _] -> [_ w435]
      tunnel: w430 -> [_ w440]
      tunnel: [_ w481] -> w428
      tunnel: [_ w480] -> w427
      tunnel: [_ w479] -> w426
      tunnel: w432 -> [_ w439]
      tunnel: w431 -> [_ w438]
      tunnel: [_ w435] -> w429
      frame #0 {
      }
      frame #1 {
        w441 = T4 0 items=["Current", "Voltage"] ("measurement type")
        n207 = Not(x=w435) -> (.not. x?=w454:bool)
        n208 = And(x=w454, y="Питание") -> (x .and. y?=w436:bool)
        n209 = call <instrlib>:"niDCPower Configure Current Limit.vi"("current limit"="ADC_curlim", "channel name"="0", "instrument handle"=w439) -> ("instrument handle out"=w516:refnum<k15>)  [unwired: 7 in, 1 out]
        n210 = call <instrlib>:"niDCPower Configure Current Limit.vi"("current limit"="STAB_curlim", "channel name"="1", "instrument handle"=w439) -> ("instrument handle out"=w517:refnum<k15>)  [unwired: 7 in, 1 out]
        n211 = call <instrlib>:"niDCPower Configure Current Limit.vi"("current limit"="RD_curlim", "channel name"="1", "instrument handle"=w438) -> ("instrument handle out"=w518:refnum<k15>)  [unwired: 7 in, 1 out]
        n212 = call <instrlib>:"niDCPower Configure Current Limit.vi"("current limit"="PH_LOW_curlim", "channel name"="2", "instrument handle"=w438) -> ("instrument handle out"=w519:refnum<k15>)  [unwired: 7 in, 1 out]
        n213 = call <instrlib>:"niDCPower Configure Current Limit.vi"("current limit"="2V_curlim", "channel name"="0", "instrument handle"=w440) -> ("instrument handle out"=w520:refnum<k15>)  [unwired: 7 in, 1 out]
        n214 = call <instrlib>:"niDCPower Configure Current Limit.vi"("current limit"="DD_curlim", "channel name"="1", "instrument handle"=w440) -> ("instrument handle out"=w521:refnum<k15>)  [unwired: 7 in, 1 out]
        n215 = call <instrlib>:"niDCPower Configure Current Limit.vi"("current limit"="PS_LOW_curlim", "channel name"="2", "instrument handle"=w440) -> ("instrument handle out"=w447:refnum<k15>)  [unwired: 7 in, 1 out]
        n216 = call <instrlib>:"niDCPower Configure Current Limit.vi"("current limit"="-15_curlim", "channel name"="2", "instrument handle"=w439) -> ("instrument handle out"=w461:refnum<k15>)  [unwired: 7 in, 1 out]
        n217 = call <instrlib>:"niDCPower Configure Current Limit.vi"("current limit"="1V_curlim", "channel name"="0", "instrument handle"=w438) -> ("instrument handle out"=w472:refnum<k15>)  [unwired: 7 in, 1 out]
        n218 = call <instrlib>:"niDCPower Configure Voltage Level.vi"("voltage level"="RD, V", "channel name"="1", "instrument handle"=w518) -> ("error out"=w499:errorcluster, "instrument handle out"=w496:refnum<k15>)  [unwired: 7 in]
        n219 = call <instrlib>:"niDCPower Configure Voltage Level.vi"("voltage level"="PH_LOW, V", "channel name"="2", "instrument handle"=w519) -> ("error out"=w498:errorcluster, "instrument handle out"=w497:refnum<k15>)  [unwired: 7 in]
        n220 = call <instrlib>:"niDCPower Configure Voltage Level.vi"("voltage level"="2V", "channel name"="0", "instrument handle"=w520) -> ("error out"=w508:errorcluster, "instrument handle out"=w511:refnum<k15>)  [unwired: 7 in]
        n221 = call <instrlib>:"niDCPower Configure Voltage Level.vi"("voltage level"="DD, V", "channel name"="1", "instrument handle"=w521) -> ("error out"=w509:errorcluster, "instrument handle out"=w510:refnum<k15>)  [unwired: 7 in]
        n222 = call <instrlib>:"niDCPower Configure Voltage Level.vi"("voltage level"="PS_LOW, V", "channel name"="2", "instrument handle"=w447) -> ("error out"=w450:errorcluster, "instrument handle out"=w449:refnum<k15>)  [unwired: 7 in]
        n223 = call <instrlib>:"niDCPower Configure Voltage Level.vi"("voltage level"="ADC, V", "channel name"="0", "instrument handle"=w516) -> ("error out"=w486:errorcluster, "instrument handle out"=w489:refnum<k15>)  [unwired: 7 in]
        n224 = call <instrlib>:"niDCPower Configure Voltage Level.vi"("voltage level"="STAB, V", "channel name"="1", "instrument handle"=w517) -> ("error out"=w487:errorcluster, "instrument handle out"=w488:refnum<k15>)  [unwired: 7 in]
        n225 = call <instrlib>:"niDCPower Configure Voltage Level.vi"("voltage level"="1V", "channel name"="0", "instrument handle"=w472) -> ("error out"=w476:errorcluster, "instrument handle out"=w477:refnum<k15>)  [unwired: 7 in]
        n226 = call <instrlib>:"niDCPower Configure Voltage Level.vi"("voltage level"="-15, V", "channel name"="2", "instrument handle"=w461) -> ("error out"=w464:errorcluster, "instrument handle out"=w463:refnum<k15>)  [unwired: 7 in]
        n227 = call <instrlib>:"niDCPower Configure Output Enabled.vi"("error in (no error)"=w499, "output enabled"=w436, "channel name"="1", "instrument handle"=w496) -> ("error out"=w545:errorcluster, "instrument handle out"=w538:refnum<k15>)  [unwired: 6 in]
        n228 = call <instrlib>:"niDCPower Configure Output Enabled.vi"("error in (no error)"=w498, "output enabled"=w436, "channel name"="2", "instrument handle"=w497) -> ("error out"=w540:errorcluster, "instrument handle out"=w539:refnum<k15>)  [unwired: 6 in]
        n229 = call <instrlib>:"niDCPower Configure Output Enabled.vi"("error in (no error)"=w508, "output enabled"=w436, "channel name"="0", "instrument handle"=w511) -> ("error out"=w542:errorcluster, "instrument handle out"=w541:refnum<k15>)  [unwired: 6 in]
        n230 = call <instrlib>:"niDCPower Configure Output Enabled.vi"("error in (no error)"=w509, "output enabled"=w436, "channel name"="1", "instrument handle"=w510) -> ("error out"=w543:errorcluster, "instrument handle out"=w544:refnum<k15>)  [unwired: 6 in]
        n231 = call <instrlib>:"niDCPower Configure Output Enabled.vi"("error in (no error)"=w450, "output enabled"=w436, "channel name"="2", "instrument handle"=w449) -> ("error out"=w444:errorcluster, "instrument handle out"=w443:refnum<k15>)  [unwired: 6 in]
        n232 = call <instrlib>:"niDCPower Configure Output Enabled.vi"("error in (no error)"=w486, "output enabled"=w436, "channel name"="0", "instrument handle"=w489) -> ("error out"=w529:errorcluster, "instrument handle out"=w528:refnum<k15>)  [unwired: 6 in]
        n233 = call <instrlib>:"niDCPower Configure Output Enabled.vi"("error in (no error)"=w487, "output enabled"=w436, "channel name"="1", "instrument handle"=w488) -> ("error out"=w530:errorcluster, "instrument handle out"=w531:refnum<k15>)  [unwired: 6 in]
        n234 = call <instrlib>:"niDCPower Configure Output Enabled.vi"("error in (no error)"=w476, "output enabled"=w436, "channel name"="0", "instrument handle"=w477) -> ("error out"=w468:errorcluster, "instrument handle out"=w469:refnum<k15>)  [unwired: 6 in]
        n235 = call <instrlib>:"niDCPower Configure Output Enabled.vi"("error in (no error)"=w464, "output enabled"=w436, "channel name"="2", "instrument handle"=w463) -> ("error out"=w459:errorcluster, "instrument handle out"=w458:refnum<k15>)  [unwired: 6 in]
        n236 = call <instrlib>:"niDCPower Measure.vi"("error in (no error)"=w529, "measurement type"=w441, "channel name"="0", "instrument handle"=w528) -> ("measurement"=→"ADC_cur":dbl, "instrument handle out"=w481:refnum<k15>)  [unwired: 5 in, 1 out]
        n237 = call <instrlib>:"niDCPower Measure.vi"("error in (no error)"=w530, "measurement type"=w441, "channel name"="1", "instrument handle"=w531) -> ("measurement"=→"STAB_cur":dbl)  [unwired: 5 in, 2 out]
        n238 = call <instrlib>:"niDCPower Measure.vi"("error in (no error)"=w459, "measurement type"=w441, "channel name"="2", "instrument handle"=w458) -> ("measurement"=→"-15_cur":dbl)  [unwired: 5 in, 2 out]
        n239 = call <instrlib>:"niDCPower Measure.vi"("error in (no error)"=w545, "measurement type"=w441, "channel name"="1", "instrument handle"=w538) -> ("measurement"=→"RD_cur":dbl, "instrument handle out"=w480:refnum<k15>)  [unwired: 5 in, 1 out]
        n240 = call <instrlib>:"niDCPower Measure.vi"("error in (no error)"=w540, "measurement type"=w441, "channel name"="2", "instrument handle"=w539) -> ("measurement"=→"PH_LOW_cur":dbl)  [unwired: 5 in, 2 out]
        n241 = call <instrlib>:"niDCPower Measure.vi"("error in (no error)"=w468, "measurement type"=w441, "channel name"="0", "instrument handle"=w469) -> ("measurement"=→"1V_cur":dbl)  [unwired: 5 in, 2 out]
        n242 = call <instrlib>:"niDCPower Measure.vi"("error in (no error)"=w542, "measurement type"=w441, "channel name"="0", "instrument handle"=w541) -> ("measurement"=→"2V_cur":dbl, "instrument handle out"=w479:refnum<k15>)  [unwired: 5 in, 1 out]
        n243 = call <instrlib>:"niDCPower Measure.vi"("error in (no error)"=w543, "measurement type"=w441, "channel name"="1", "instrument handle"=w544) -> ("measurement"=→"DD_cur":dbl)  [unwired: 5 in, 2 out]
        n244 = call <instrlib>:"niDCPower Measure.vi"("error in (no error)"=w444, "measurement type"=w441, "channel name"="2", "instrument handle"=w443) -> ("measurement"=→"PS_LOW_cur":dbl)  [unwired: 5 in, 2 out]
      }
    }
    n245 = Wait (ms)(milliseconds to wait=u32 1) -> ()  [unwired: 1 out]
  }
  n246 = while {
    tunnel: w1 -> [w562]
    shift-right: ["文韧 世男!"] -> _
    shift-left: _ -> [w558]
    stop <- w563 stop-if-true
    # "Запрос кадра"
    n247 = local read "Линейки"() -> (w561:bool)
    n248 = local read "Питание"() -> (w560:bool)
    n249 = Greater?(x="文韧 世男!", y=w558) -> (0:w555:bool)
    n250 = Or(x=w555, y="НЕПРЕРЫВНО") -> (x .or. y?=w556:bool)
    n251 = Compound Arithmetic op=AND(w556, w561, w560) -> (w559:bool)
    n252 = case shown="True" w559 {
      tunnel: w562 -> [_ w565]
      frame False {
        n253 = Wait (ms)(milliseconds to wait=u32 1) -> ()  [unwired: 1 out]
      }
      frame True {
        n254 = stacked-sequence {
          seq-local: [_ w577 _ _ _ _] -> [_ _ w647 _ _ _]
          seq-local: [_ _ w657 _ _ _] -> [_ _ _ w689 _ _]
          seq-local: [_ _ _ w688 _ _] -> [_ _ _ _ w693 _]
          tunnel: w565 -> [w567 w578 _ _ _ _]
          frame #0 {
            n255 = xnode "Invoke Method"("FPGA VI Reference In"=w567, "Number of Elements"=u32 0, "Timeout (ms)"=0) -> ("FPGA VI Reference Out"=w572:refnum<k20>, "Elements Remaining"=w571:u32)  [unwired: 1 in, 2 out]
            n256 = local write "БД"(0 ("БД")) -> ()
            n257 = xnode "Invoke Method"("FPGA VI Reference In"=w572, "Number of Elements"=w571, "Timeout (ms)"=0) -> ()  [unwired: 1 in, 4 out]
          }
          frame #1 {
            n258 = for {
              N: "Усреднение" -> [_]
              tunnel: w578 -> [w586]
              shift-right: [w583] -> w576
              shift-left: u64[] array[96800 elements] -> [w584]
              n259 = stacked-sequence {
                seq-local: [_ w591 _ _] -> [_ _ w603 _]
                tunnel: w586 -> [w588 w590 w597 _]
                tunnel: [_ _ w599 _] -> w585
                frame #0 {
                  n260 = xnode "Read/Write Control"("FPGA VI Reference In"=w588, "Кадр в FIFO"=TRUE) -> ()  [unwired: 1 in, 2 out]
                  n261 = Wait (ms)(milliseconds to wait=u32 300) -> ()  [unwired: 1 out]
                }
                frame #1 {
                  n262 = xnode "Invoke Method"("FPGA VI Reference In"=w590, "Number of Elements"=u32 0, "Timeout (ms)"=0) -> ("FPGA VI Reference Out"=w593:refnum<k20>, "Elements Remaining"=w592:u32)  [unwired: 1 in, 2 out]
                  n263 = xnode "Invoke Method"("FPGA VI Reference In"=w593, "Number of Elements"=w592, "Timeout (ms)"=0) -> ("Data"=w591:u8[])  [unwired: 1 in, 3 out]
                }
                frame #2 {
                  # "L"
                  # "H"
                  n264 = Decimate 1D Array(w603) -> (w602:u8[], w601:u8[])
                  n265 = for {
                    N: 96800 -> [_]
                    tunnel: w602 -> [w613]
                    tunnel: w601 -> [w612]
                    tunnel: [w604] -> w599 mode=indexing
                    i -> [w611]
                    n266 = Index Array(array=w612, index=w611) -> (element=w609:u8)
                    n267 = Index Array(array=w613, index=w611) -> (element=w610:u8)
                    n268 = To Unsigned Word Integer(number=w609) -> (unsigned 16bit integer=w605:u16)
                    n269 = To Unsigned Word Integer(number=w610) -> (unsigned 16bit integer=w608:u16)
                    n270 = Multiply(x=w608, y=u16 256) -> (x*y=w606:u16)
                    n271 = Add(x=w606, y=w605) -> (x+y=w604:u16)
                  }
                  n272 = xnode "Read/Write Control"("FPGA VI Reference In"=w597, "Кадр в FIFO"=FALSE) -> ()  [unwired: 1 in, 2 out]
                }
                frame #3 {
                  n273 = Wait (ms)(milliseconds to wait=u32 300) -> ()  [unwired: 1 out]
                }
              }
              n274 = Add(x=w585, y=w584) -> (x+y=w583:u64[])
            }
            n275 = local write "FRAME_OK"(FALSE ("FRAME_OK")) -> ()
            n276 = for {
              tunnel: w576 -> [w582] mode=indexing
              tunnel: "Усреднение" -> [w581]
              tunnel: [w579] -> w577 mode=indexing
              n277 = Divide(x=w582, y=w581) -> (x/y=w580:dbl)
              n278 = To Unsigned Word Integer(number=w580) -> (unsigned 16bit integer=w579:u16)
            }
          }
          frame #2 {
            w621 = 840 ("length")
            w622 = 62 ("length")
            w652 = 4 ("length")
            w651 = 8 ("length")
            n279 = Multiply(x=w622, y=w621) -> (x*y=w625:i32)
            n280 = Multiply(x=w647, y="ISO") -> (x*y=w646:dbl[])
            n281 = To Unsigned Word Integer(number=w646) -> (unsigned 16bit integer=w645:u16[])
            n282 = for {
              N: 110 -> [_]
              tunnel: [w684] -> w616 mode=indexing
              shift-right: [w683] -> _
              shift-left: w645 -> [w687]
              n283 = Delete From Array(array=w687, length=880, index=0) -> (deleted portion=w684:u16[], array with subset deleted=w683:u16[])
            }
            "FRAME" <- w616
            n284 = Array Subset(array=w616, index (row)=2 ("index"), length (row)=w622, index (col)=26 ("index"), length (col)=w621) -> (w619:u16[][])
            n285 = Reshape Array(w619, w625) -> (w618:u16[])
            n286 = for {
              tunnel: w618 -> [w661] mode=indexing
              shift-right: [w659] -> w617
              shift-left: u64 0 -> [w660]
              n287 = Add(x=w661, y=w660) -> (x+y=w659:u64)
            }
            n288 = for {
              tunnel: w616 -> [w679] mode=indexing
              tunnel: [w678] -> w657 mode=indexing
              n289 = for {
                N: 880 -> [_]
                tunnel: [w682] -> w678 mode=indexing
                tunnel: w679 -> [w681] mode=indexing
                n290 = Bundle(w681, w681, w681, w681) -> (w682:cluster{u16, u16, u16, u16})  [unwired: 1 in]
              }
            }
            "OUT" <- w657
            n291 = Divide(x=w617, y=w625) -> (x/y=w615:dbl)
            n292 = Array Subset(array=w616, index (row)=2 ("index"), length (row)=62 ("length"), index (col)=26 ("index"), length (col)=840 ("length")) -> (w629:u16[][])
            n293 = Multiply(x=w651, y=w652) -> (x*y=w636:i32)
            n294 = Array Subset(array=w616, index (row)=101 ("index"), length (row)=w651, index (col)=9 ("index"), length (col)=w652) -> (w654:u16[][])
            n295 = Array Subset(array=w616, index (row)=101 ("index"), length (row)=8 ("length"), index (col)=9 ("index"), length (col)=4 ("length")) -> (w643:u16[][])
            n296 = Reshape Array(w654, w636) -> (w655:u16[])
            n297 = Reshape Array(w643, w636) -> (w639:u16[])
            n298 = Multiply(x=5.0, y=w615) -> (x*y=w627:dbl)
            n299 = for {
              tunnel: w629 -> [w663] mode=indexing
              tunnel: w627 -> [w662]
              n300 = for {
                tunnel: w663 -> [w666] mode=indexing
                tunnel: w662 -> [w664]
                n301 = Greater Or Equal?(x=w666, y=w664) -> (x >= y?=w665:bool)
                n302 = case shown="True" w665 {
                  frame False {
                  }
                  frame True {
                    n303 = local read "БД"() -> (w668:i32)
                    n304 = Increment(x=w668) -> (x+1=→"БД":i32)
                  }
                }
              }
            }
            n305 = for {
              tunnel: w655 -> [w677] mode=indexing
              shift-right: [w675] -> w656
              shift-left: u64 0 -> [w676]
              n306 = Add(x=w677, y=w676) -> (x+y=w675:u64)
            }
            n307 = Divide(x=w656, y=w636) -> (x/y=w626:dbl)
            "Среднее" <- w626
            n308 = for {
              tunnel: w626 -> [w673]
              tunnel: w639 -> [w674] mode=indexing
              shift-right: [w669] -> w644
              shift-left: 0.0 -> [w671]
              n309 = Subtract(x=w674, y=w673) -> (x-y=w672:dbl)
              n310 = Square(x=w672) -> (x^2=w670:dbl)
              n311 = Add(x=w670, y=w671) -> (x+y=w669:dbl)
            }
            n312 = Divide(x=w644, y=w636) -> (x/y=w635:dbl)
            n313 = Square Root(x=w635) -> (sqrt(x)=→"СКО":dbl)
          }
          frame #3 {
            w690 = T5 6 items=["Grayscale (U8)", "Grayscale (I16)", "Grayscale (SGL)", "Complex (CSG)", "RGB (U32)", "HSL (U32)", "RGB (U64)"] ("Image Type")
            n314 = call "IMAQ Create"("Image Name"="FPZC", "Image Type"=w690) -> ("New Image"=w692:T1)  [unwired: 3 in, 1 out]
            n315 = call "IMAQ ArrayToColorImage"("Image"=w692, "Image Pixels (U64)"=w689) -> ("Image Out"=w688:T1)  [unwired: 3 in, 1 out]
            "Image" <- w688
          }
          frame #4 {
            n316 = case shown="True" "Запись Кадра" {
              tunnel: w693 -> [_ w698]
              frame False {
              }
              frame True {
                w703 = i16 0 ("precision (6)")
                w697 = "_"
                n317 = local read "Между кадрами, мс"() -> (w715:u8)
                n318 = local read "Номер образца"() -> (w709:string)
                n319 = Concatenate Strings("Образец_" ("string"), w709) -> (w704:string)
                n320 = Get Date/Time In Seconds() -> (seconds since 1Jan1904=w712:timestamp)
                n321 = Build Path(base path="Frames", name or relative path=w704) -> (appended path=w708:path)
                n322 = Number To Fractional String(number=w715, width (-)=w703, precision (6)=w703) -> (F-format string=w716:string)  [unwired: 1 in]
                n323 = Format Date/Time String(time format string (%c)="%H.%M.%S", seconds (now)=w712) -> (date/time string=w714:string)  [unwired: 1 in]
                n324 = call <vilib>:"Check if File or Folder Exists.vi"("path"=w708) -> ("file or folder exists?"=w707:bool, "dup path"=w706:path)  [unwired: 8 in, 1 out]
                n325 = case shown="False" w707 {
                  tunnel: w706 -> [w719 w720]
                  tunnel: [w718 w720] -> w713
                  frame False {
                    n326 = Create Folder(path (use dialog)=w719) -> (created path=w718:path)  [unwired: 2 in, 2 out]
                  }
                  frame True {
                  }
                }
                n327 = Concatenate Strings(w714, w697, "Тн=" ("string"), w716, "мс_" ("string"), "ПРИМЕЧАНИЕ", w697, "Какая фотка?", ".tiff" ("element")) -> (w710:string)
                n328 = Build Path(base path=w713, name or relative path=w710) -> (appended path=w711:path)
                n329 = call-poly "IMAQ Write File 2"("File Path"=w711, "Image"=w698) -> ()  [unwired: 8 in, 2 out]
              }
            }
          }
          frame #5 {
            "FRAME_OK" <- TRUE
          }
        }
      }
    }
    n330 = local read "Стоп"() -> (w563:bool)
  }
  n331 = while {
    tunnel: w1 -> [w727]
    shift-right: ["Прошить АЦП"] -> _
    shift-left: FALSE -> [w726]
    stop <- w728 stop-if-true
    n332 = Greater?(x="Прошить АЦП", y=w726) -> (0:w724:bool)
    n333 = local read "Питание"() -> (w722:bool)
    n334 = And(x=w722, y=w724) -> (x .and. y?=w723:bool)
    n335 = case shown="True" w723 {
      tunnel: w727 -> [_ w730]
      frame False {
        n336 = Wait (ms)(milliseconds to wait=u32 1) -> ()  [unwired: 1 out]
      }
      frame True {
        n337 = stacked-sequence {
          tunnel: w730 -> [w756 w796 w810 w839 w883 w893 w918 w951 _]
          frame #0 {
            w752 = TRUE ("element")
            w753 = FALSE
            # "8"
            # "0"
            # "Configuration"
            n338 = xnode "Read/Write Control"("FPGA VI Reference In"=w756, "Enum"=T6."Configuration") -> ("FPGA VI Reference Out"=w743:refnum<k20>)  [unwired: 1 in, 1 out]
            n339 = xnode "Read/Write Control"("FPGA VI Reference In"=w733, "Read(T)/Write(F)"=TRUE) -> ("FPGA VI Reference Out"=w739:refnum<k20>, "error out"=w738:errorcluster)  [unwired: 1 in]
            n340 = case shown="\"3CH\", Default" "3CH/1CH" {
              tunnel: [TRUE FALSE] -> w751
              frame "3CH", Default {
              }
              frame "1CH" {
              }
            }
            n341 = case shown="\"4V\"" "2/4 V" {
              tunnel: [FALSE TRUE] -> w749
              frame "2V", Default {
              }
              frame "4V" {
              }
            }
            n342 = xnode "Read/Write Control"("FPGA VI Reference In"=w743, "Read(T)/Write(F)"=FALSE) -> ("FPGA VI Reference Out"=w741:refnum<k20>)  [unwired: 1 in, 1 out]
            n343 = flat-sequence {
              tunnel: w739 -> [w768]
              tunnel: w738 -> [w767]
              tunnel: [w766] -> w737
              tunnel: [w765] -> w736
              frame #0 {
                n344 = xnode "Read/Write Control"("FPGA VI Reference In"=w768, "error in"=w767, "Конфигурация"=TRUE) -> ("FPGA VI Reference Out"=w766:refnum<k20>, "error out"=w765:errorcluster)
                n345 = Wait (ms)(milliseconds to wait=u32 10) -> ()  [unwired: 1 out]
              }
            }
            n346 = Build Array(w753, w753, w753, w752, w752, w751, w752, w749, FALSE) -> (w754:bool[])
            n347 = Reverse 1D Array(array=w754) -> (reversed array=w746:bool[])
            n348 = xnode "Read/Write Control"("FPGA VI Reference In"=w741, "Write Data"=w746) -> ("FPGA VI Reference Out"=w745:refnum<k20>)  [unwired: 1 in, 1 out]
            n349 = flat-sequence {
              tunnel: w737 -> [w762]
              tunnel: w736 -> [w761]
              tunnel: [w759] -> w735
              tunnel: [w758] -> w734
              frame #0 {
                n350 = xnode "Read/Write Control"("FPGA VI Reference In"=w762, "error in"=w761, "Конфигурация"=FALSE) -> ("FPGA VI Reference Out"=w759:refnum<k20>, "error out"=w758:errorcluster)
                n351 = Wait (ms)(milliseconds to wait=u32 10) -> ()  [unwired: 1 out]
              }
            }
            n352 = flat-sequence {
              tunnel: w745 -> [w776]
              tunnel: [w774] -> w744
              frame #0 {
                n353 = xnode "Read/Write Control"("FPGA VI Reference In"=w776, "Конфигурация"=TRUE) -> ("FPGA VI Reference Out"=w774:refnum<k20>)  [unwired: 1 in, 1 out]
                n354 = Wait (ms)(milliseconds to wait=u32 10) -> ()  [unwired: 1 out]
              }
            }
            n355 = local write "АЦП прошит!"(FALSE ("АЦП прошит!")) -> ()
            n356 = xnode "Read/Write Control"("FPGA VI Reference In"=w735, "error in"=w734) -> ("READ"=→"Configuration":bool[])  [unwired: 2 out]
            n357 = flat-sequence {
              tunnel: w744 -> [w772]
              tunnel: [w770] -> w733
              frame #0 {
                n358 = xnode "Read/Write Control"("FPGA VI Reference In"=w772, "Конфигурация"=FALSE) -> ("FPGA VI Reference Out"=w770:refnum<k20>)  [unwired: 1 in, 1 out]
                n359 = Wait (ms)(milliseconds to wait=u32 10) -> ()  [unwired: 1 out]
              }
            }
          }
          frame #1 {
            # "GREEN_OFFSET"
            n360 = case shown="\"-\", Default" "+/- OUT2" {
              tunnel: [TRUE FALSE] -> w783
              frame "-", Default {
              }
              frame "+" {
              }
            }
            n361 = Quotient & Remainder(x="Смещение, до 300_OUT2", y=1.171875) -> (floor(x/y)=w788:dbl)  [unwired: 1 out]
            n362 = xnode "Read/Write Control"("FPGA VI Reference In"=w796, "Enum"=T6."GREEN OFF" ("OFFSET")) -> ("FPGA VI Reference Out"=w795:refnum<k20>, "error out"=w794:errorcluster)  [unwired: 1 in]
            n363 = Subtract(x=w788, y=1.0) -> (x-y=w785:dbl)
            n364 = To Unsigned Byte Integer(number=w785) -> (unsigned 8bit integer=w784:u8)
            n365 = xnode "Read/Write Control"("FPGA VI Reference In"=w795, "error in"=w794, "Read(T)/Write(F)"=FALSE) -> ("FPGA VI Reference Out"=w793:refnum<k20>)  [unwired: 1 out]
            n366 = Number To Boolean Array(number=w784) -> (Boolean array=w782:bool[])
            n367 = Reverse 1D Array(array=w782) -> (reversed array=w781:bool[])
            n368 = Build Array (concatenate)(w783, w781) -> (w786:bool[])
            n369 = xnode "Read/Write Control"("FPGA VI Reference In"=w793, "Write Data"=w786) -> ("FPGA VI Reference Out"=w798:refnum<k20>)  [unwired: 1 in, 1 out]
            n370 = flat-sequence {
              tunnel: w798 -> [w809]
              tunnel: [w807] -> w797
              frame #0 {
                n371 = xnode "Read/Write Control"("FPGA VI Reference In"=w809, "Конфигурация"=TRUE) -> ("FPGA VI Reference Out"=w807:refnum<k20>)  [unwired: 1 in, 1 out]
                n372 = Wait (ms)(milliseconds to wait=u32 10) -> ()  [unwired: 1 out]
              }
            }
            n373 = flat-sequence {
              tunnel: w797 -> [w805]
              tunnel: [w803] -> _
              frame #0 {
                n374 = xnode "Read/Write Control"("FPGA VI Reference In"=w805, "Конфигурация"=FALSE) -> ("FPGA VI Reference Out"=w803:refnum<k20>)  [unwired: 1 in, 1 out]
                n375 = Wait (ms)(milliseconds to wait=u32 10) -> ()  [unwired: 1 out]
              }
            }
          }
          frame #2 {
            # "RED_OFFSET"
            n376 = case shown="\"-\", Default" "+/- OUT3" {
              tunnel: [TRUE FALSE] -> w826
              frame "-", Default {
              }
              frame "+" {
              }
            }
            n377 = Quotient & Remainder(x="Смещение, до 300_OUT3", y=1.171875) -> (floor(x/y)=w821:dbl)  [unwired: 1 out]
            n378 = xnode "Read/Write Control"("FPGA VI Reference In"=w810, "Enum"=T6."RED OFF" ("OFFSET")) -> ("FPGA VI Reference Out"=w817:refnum<k20>, "error out"=w818:errorcluster)  [unwired: 1 in]
            n379 = Subtract(x=w821, y=1.0) -> (x-y=w824:dbl)
            n380 = To Unsigned Byte Integer(number=w824) -> (unsigned 8bit integer=w825:u8)
            n381 = xnode "Read/Write Control"("FPGA VI Reference In"=w817, "error in"=w818, "Read(T)/Write(F)"=FALSE) -> ("FPGA VI Reference Out"=w819:refnum<k20>)  [unwired: 1 out]
            n382 = Number To Boolean Array(number=w825) -> (Boolean array=w827:bool[])
            n383 = Reverse 1D Array(array=w827) -> (reversed array=w828:bool[])
            n384 = Build Array (concatenate)(w826, w828) -> (w823:bool[])
            n385 = xnode "Read/Write Control"("FPGA VI Reference In"=w819, "Write Data"=w823) -> ("FPGA VI Reference Out"=w815:refnum<k20>)  [unwired: 1 in, 1 out]
            n386 = flat-sequence {
              tunnel: w815 -> [w838]
              tunnel: [w836] -> w816
              frame #0 {
                n387 = xnode "Read/Write Control"("FPGA VI Reference In"=w838, "Конфигурация"=TRUE) -> ("FPGA VI Reference Out"=w836:refnum<k20>)  [unwired: 1 in, 1 out]
                n388 = Wait (ms)(milliseconds to wait=u32 10) -> ()  [unwired: 1 out]
              }
            }
            n389 = flat-sequence {
              tunnel: w816 -> [w834]
              tunnel: [w832] -> _
              frame #0 {
                n390 = xnode "Read/Write Control"("FPGA VI Reference In"=w834, "Конфигурация"=FALSE) -> ("FPGA VI Reference Out"=w832:refnum<k20>)  [unwired: 1 in, 1 out]
                n391 = Wait (ms)(milliseconds to wait=u32 10) -> ()  [unwired: 1 out]
              }
            }
          }
          frame #3 {
            # "BLUE_OFFSET"
            n392 = case shown="\"-\", Default" "+/- OUT1" {
              tunnel: [TRUE FALSE] -> w855
              frame "-", Default {
              }
              frame "+" {
              }
            }
            n393 = Quotient & Remainder(x="Смещение, до 300_OUT1", y=1.171875) -> (floor(x/y)=w850:dbl)  [unwired: 1 out]
            n394 = xnode "Read/Write Control"("FPGA VI Reference In"=w839, "Enum"=T6."BLUE OFF" ("OFFSET")) -> ("FPGA VI Reference Out"=w846:refnum<k20>, "error out"=w847:errorcluster)  [unwired: 1 in]
            n395 = Subtract(x=w850, y=1.0) -> (x-y=w853:dbl)
            n396 = To Unsigned Byte Integer(number=w853) -> (unsigned 8bit integer=w854:u8)
            n397 = xnode "Read/Write Control"("FPGA VI Reference In"=w846, "error in"=w847, "Read(T)/Write(F)"=FALSE) -> ("FPGA VI Reference Out"=w848:refnum<k20>)  [unwired: 1 out]
            n398 = Number To Boolean Array(number=w854) -> (Boolean array=w856:bool[])
            n399 = Reverse 1D Array(array=w856) -> (reversed array=w857:bool[])
            n400 = Build Array (concatenate)(w855, w857) -> (w852:bool[])
            n401 = xnode "Read/Write Control"("FPGA VI Reference In"=w848, "Write Data"=w852) -> ("FPGA VI Reference Out"=w844:refnum<k20>)  [unwired: 1 in, 1 out]
            n402 = flat-sequence {
              tunnel: w844 -> [w867]
              tunnel: [w865] -> w845
              frame #0 {
                n403 = xnode "Read/Write Control"("FPGA VI Reference In"=w867, "Конфигурация"=TRUE) -> ("FPGA VI Reference Out"=w865:refnum<k20>)  [unwired: 1 in, 1 out]
                n404 = Wait (ms)(milliseconds to wait=u32 10) -> ()  [unwired: 1 out]
              }
            }
            n405 = flat-sequence {
              tunnel: w845 -> [w863]
              tunnel: [w861] -> _
              frame #0 {
                n406 = xnode "Read/Write Control"("FPGA VI Reference In"=w863, "Конфигурация"=FALSE) -> ("FPGA VI Reference Out"=w861:refnum<k20>)  [unwired: 1 in, 1 out]
                n407 = Wait (ms)(milliseconds to wait=u32 10) -> ()  [unwired: 1 out]
              }
            }
          }
          frame #4 {
            w878 = FALSE
            # "GREEN PGA"
            n408 = Decrement(x="Усиление (до 6)_OUT2") -> (x-1=w870:u8)
            n409 = Multiply(x=w870, y=378) -> (x*y=w872:i32)
            n410 = Multiply(x="Усиление (до 6)_OUT2", y=5) -> (x*y=w875:i32)
            n411 = xnode "Read/Write Control"("FPGA VI Reference In"=w883, "Enum"=T6."GREEN PGA" ("PGA")) -> ("FPGA VI Reference Out"=w881:refnum<k20>)  [unwired: 1 in, 1 out]
            n412 = Divide(x=w872, y=w875) -> (x/y=w876:dbl)
            n413 = Number To Boolean Array(number=w876) -> (Boolean array=w869:bool[])
            n414 = xnode "Read/Write Control"("FPGA VI Reference In"=w881, "Read(T)/Write(F)"=FALSE) -> ("FPGA VI Reference Out"=w880:refnum<k20>)  [unwired: 1 in, 1 out]
            n415 = Build Array (concatenate)(w878, w878, w878, w869) -> (w877:bool[])
            n416 = xnode "Read/Write Control"("FPGA VI Reference In"=w880, "Write Data"=w877) -> ("FPGA VI Reference Out"=w882:refnum<k20>)  [unwired: 1 in, 1 out]
            n417 = flat-sequence {
              tunnel: [w891] -> w884
              tunnel: w882 -> [w890]
              frame #0 {
                n418 = xnode "Read/Write Control"("FPGA VI Reference In"=w890, "Конфигурация"=TRUE) -> ("FPGA VI Reference Out"=w891:refnum<k20>)  [unwired: 1 in, 1 out]
                n419 = Wait (ms)(milliseconds to wait=u32 10) -> ()  [unwired: 1 out]
              }
            }
            n420 = flat-sequence {
              tunnel: w884 -> [w888]
              tunnel: [w886] -> _
              frame #0 {
                n421 = xnode "Read/Write Control"("FPGA VI Reference In"=w888, "Конфигурация"=FALSE) -> ("FPGA VI Reference Out"=w886:refnum<k20>)  [unwired: 1 in, 1 out]
                n422 = Wait (ms)(milliseconds to wait=u32 10) -> ()  [unwired: 1 out]
              }
            }
          }
          frame #5 {
            w896 = FALSE
            # "BLUE PGA"
            n423 = Decrement(x="Усиление (до 6)_OUT1") -> (x-1=w900:u8)
            n424 = Multiply(x=w900, y=378) -> (x*y=w901:i32)
            n425 = Multiply(x="Усиление (до 6)_OUT1", y=5) -> (x*y=w903:i32)
            n426 = xnode "Read/Write Control"("FPGA VI Reference In"=w893, "Enum"=T6."BLUE PGA" ("PGA")) -> ("FPGA VI Reference Out"=w907:refnum<k20>)  [unwired: 1 in, 1 out]
            n427 = Divide(x=w901, y=w903) -> (x/y=w904:dbl)
            n428 = Number To Boolean Array(number=w904) -> (Boolean array=w899:bool[])
            n429 = xnode "Read/Write Control"("FPGA VI Reference In"=w907, "Read(T)/Write(F)"=FALSE) -> ("FPGA VI Reference Out"=w906:refnum<k20>)  [unwired: 1 in, 1 out]
            n430 = Build Array (concatenate)(w896, w896, w896, w899) -> (w905:bool[])
            n431 = xnode "Read/Write Control"("FPGA VI Reference In"=w906, "Write Data"=w905) -> ("FPGA VI Reference Out"=w908:refnum<k20>)  [unwired: 1 in, 1 out]
            n432 = flat-sequence {
              tunnel: [w916] -> w909
              tunnel: w908 -> [w915]
              frame #0 {
                n433 = xnode "Read/Write Control"("FPGA VI Reference In"=w915, "Конфигурация"=TRUE) -> ("FPGA VI Reference Out"=w916:refnum<k20>)  [unwired: 1 in, 1 out]
                n434 = Wait (ms)(milliseconds to wait=u32 10) -> ()  [unwired: 1 out]
              }
            }
            n435 = flat-sequence {
              tunnel: w909 -> [w913]
              tunnel: [w911] -> _
              frame #0 {
                n436 = xnode "Read/Write Control"("FPGA VI Reference In"=w913, "Конфигурация"=FALSE) -> ("FPGA VI Reference Out"=w911:refnum<k20>)  [unwired: 1 in, 1 out]
                n437 = Wait (ms)(milliseconds to wait=u32 10) -> ()  [unwired: 1 out]
              }
            }
          }
          frame #6 {
            w929 = FALSE
            # "RED PGA"
            n438 = Decrement(x="Усиление (до 6)_OUT3") -> (x-1=w921:u8)
            n439 = Multiply(x=w921, y=378) -> (x*y=w923:i32)
            n440 = Multiply(x="Усиление (до 6)_OUT3", y=5) -> (x*y=w926:i32)
            n441 = xnode "Read/Write Control"("FPGA VI Reference In"=w918, "Enum"=T6."RED PGA" ("PGA")) -> ("FPGA VI Reference Out"=w932:refnum<k20>)  [unwired: 1 in, 1 out]
            n442 = Divide(x=w923, y=w926) -> (x/y=w927:dbl)
            n443 = Number To Boolean Array(number=w927) -> (Boolean array=w920:bool[])
            n444 = xnode "Read/Write Control"("FPGA VI Reference In"=w932, "Read(T)/Write(F)"=FALSE) -> ("FPGA VI Reference Out"=w931:refnum<k20>)  [unwired: 1 in, 1 out]
            n445 = Build Array (concatenate)(w929, w929, w929, w920) -> (w928:bool[])
            n446 = xnode "Read/Write Control"("FPGA VI Reference In"=w931, "Write Data"=w928) -> ("FPGA VI Reference Out"=w933:refnum<k20>)  [unwired: 1 in, 1 out]
            n447 = flat-sequence {
              tunnel: [w941] -> w934
              tunnel: w933 -> [w940]
              frame #0 {
                n448 = xnode "Read/Write Control"("FPGA VI Reference In"=w940, "Конфигурация"=TRUE) -> ("FPGA VI Reference Out"=w941:refnum<k20>)  [unwired: 1 in, 1 out]
                n449 = Wait (ms)(milliseconds to wait=u32 10) -> ()  [unwired: 1 out]
              }
            }
            n450 = flat-sequence {
              tunnel: w934 -> [w938]
              tunnel: [w936] -> _
              frame #0 {
                n451 = xnode "Read/Write Control"("FPGA VI Reference In"=w938, "Конфигурация"=FALSE) -> ("FPGA VI Reference Out"=w936:refnum<k20>)  [unwired: 1 in, 1 out]
                n452 = Wait (ms)(milliseconds to wait=u32 10) -> ()  [unwired: 1 out]
              }
            }
          }
          frame #7 {
            # "MUX"
            n453 = xnode "Read/Write Control"("FPGA VI Reference In"=w951, "Enum"=T6."MUX") -> ("FPGA VI Reference Out"=w945:refnum<k20>)  [unwired: 1 in, 1 out]
            n454 = case shown="\"OUT1\", Default" "Какой канал?" {
              tunnel: [bool[] [FALSE, TRUE, FALSE, FALSE, TRUE, FALSE, FALSE, FALSE, FALSE] ("MUX_register") bool[] [FALSE, TRUE, FALSE, TRUE, FALSE, FALSE, FALSE, FALSE, FALSE] ("MUX_register") bool[] [FALSE, TRUE, TRUE, FALSE, FALSE, FALSE, FALSE, FALSE, FALSE] ("MUX_register")] -> w943
              frame "OUT1", Default {
              }
              frame "OUT2" {
              }
              frame "OUT3" {
              }
            }
            n455 = xnode "Read/Write Control"("FPGA VI Reference In"=w945, "Read(T)/Write(F)"=FALSE) -> ("FPGA VI Reference Out"=w947:refnum<k20>)  [unwired: 1 in, 1 out]
            n456 = xnode "Read/Write Control"("FPGA VI Reference In"=w947, "Write Data"=w943) -> ("FPGA VI Reference Out"=w948:refnum<k20>)  [unwired: 1 in, 1 out]
            n457 = flat-sequence {
              tunnel: [w961] -> w949
              tunnel: w948 -> [w960]
              frame #0 {
                n458 = xnode "Read/Write Control"("FPGA VI Reference In"=w960, "Конфигурация"=TRUE) -> ("FPGA VI Reference Out"=w961:refnum<k20>)  [unwired: 1 in, 1 out]
                n459 = Wait (ms)(milliseconds to wait=u32 10) -> ()  [unwired: 1 out]
              }
            }
            n460 = flat-sequence {
              tunnel: w949 -> [w958]
              tunnel: [w956] -> _
              frame #0 {
                n461 = xnode "Read/Write Control"("FPGA VI Reference In"=w958, "Конфигурация"=FALSE) -> ("FPGA VI Reference Out"=w956:refnum<k20>)  [unwired: 1 in, 1 out]
                n462 = Wait (ms)(milliseconds to wait=u32 10) -> ()  [unwired: 1 out]
              }
            }
          }
          frame #8 {
            "АЦП прошит!" <- TRUE ("АЦП прошит!")
          }
        }
      }
    }
    n463 = local read "Стоп"() -> (w728:bool)
  }
  n464 = while {
    shift-right: [w966] -> _
    shift-left: _ -> [w967]
    tunnel: w5 -> [_]
    tunnel: w2 -> [w964]
    stop <- w965 stop-if-true
    n465 = stacked-sequence {
      tunnel: [_ _ _ _ w1089] -> w965
      tunnel: w967 -> [w971 _ _ _ _]
      tunnel: [w970 _ _ _ _] -> w966
      tunnel: w964 -> [_ _ _ w1054 _]
      frame #0 {
        n466 = local read "Питание"() -> (w970:bool)
        n467 = Greater?(x=w970, y=w971) -> (0:w969:bool)
        n468 = case shown="True" w969 {
          frame False {
          }
          frame True {
            n469 = flat-sequence {
              frame #0 {
                n470 = Wait (ms)(milliseconds to wait=u32 500) -> ()  [unwired: 1 out]
              }
              frame #1 {
                n471 = local write "Прошить АЦП"(TRUE ("Прошить АЦП")) -> ()
                n472 = Wait (ms)(milliseconds to wait=u32 25) -> ()  [unwired: 1 out]
              }
              frame #2 {
                n473 = local write "Прошить АЦП"(FALSE ("Прошить АЦП")) -> ()
                n474 = Wait (ms)(milliseconds to wait=u32 25) -> ()  [unwired: 1 out]
              }
            }
          }
        }
      }
      frame #1 {
        n475 = local read "Питание"() -> (w977:bool)
        n476 = case shown="True" w977 {
          frame False {
          }
          frame True {
            n477 = local read "2V_cur"() -> (w987:dbl)
            n478 = local read "2V_curlim"() -> (w986:dbl)
            n479 = local read "0,005"() -> (w981:dbl)
            n480 = local read "1V_curlim"() -> (w1002:dbl)
            n481 = local read "ADC_cur"() -> (w1016:dbl)
            n482 = local read "ADC_curlim"() -> (w1015:dbl)
            n483 = local read "0,005"() -> (w992:dbl)
            n484 = local read "1V_cur"() -> (w1003:dbl)
            n485 = Subtract(x=w1002, y=w992) -> (x-y=w1004:dbl)
            n486 = Subtract(x=w986, y=w981) -> (x-y=w990:dbl)
            n487 = Subtract(x=w1015, y="0,005") -> (x-y=w1014:dbl)
            n488 = Greater?(x=w1003, y=w1004) -> (0:→"1V":bool)
            n489 = Greater?(x=w987, y=w990) -> (0:→"2V":bool)
            n490 = Greater?(x=w1016, y=w1014) -> (0:→"ADC":bool)
            n491 = local read "RD_curlim"() -> (w999:dbl)
            n492 = local read "DD_cur"() -> (w985:dbl)
            n493 = local read "DD_curlim"() -> (w984:dbl)
            n494 = local read "RD_cur"() -> (w1000:dbl)
            n495 = local read "STAB_cur"() -> (w1011:dbl)
            n496 = local read "STAB_curlim"() -> (w1010:dbl)
            n497 = Subtract(x=w999, y=w992) -> (x-y=w998:dbl)
            n498 = Greater?(x=w1000, y=w998) -> (0:→"RD":bool)
            n499 = local read "PH_LOW_curlim"() -> (w993:dbl)
            n500 = Subtract(x=w984, y=w981) -> (x-y=w989:dbl)
            n501 = Subtract(x=w1010, y="0,005") -> (x-y=w1012:dbl)
            n502 = Greater?(x=w985, y=w989) -> (0:→"DD":bool)
            n503 = local read "PH_LOW_cur"() -> (w994:dbl)
            n504 = Greater?(x=w1011, y=w1012) -> (0:→"STAB":bool)
            n505 = local read "-15_curlim"() -> (w1006:dbl)
            n506 = local read "PS_LOW_cur"() -> (w983:dbl)
            n507 = local read "PS_LOW_curlim"() -> (w982:dbl)
            n508 = Subtract(x=w993, y=w992) -> (x-y=w995:dbl)
            n509 = local read "-15_cur"() -> (w1007:dbl)
            n510 = Greater?(x=w994, y=w995) -> (0:→"PH":bool)
            n511 = Subtract(x=w1006, y="0,005") -> (x-y=w1008:dbl)
            n512 = Greater?(x=w1007, y=w1008) -> (0:→"-15":bool)
            n513 = Subtract(x=w982, y=w981) -> (x-y=w988:dbl)
            n514 = Greater?(x=w983, y=w988) -> (0:→"PS":bool)
          }
        }
      }
      frame #2 {
        n515 = local read "ADC"() -> (w1023:bool)
        n516 = local read "STAB"() -> (w1022:bool)
        n517 = local read "-15"() -> (w1021:bool)
        n518 = local read "1V"() -> (w1020:bool)
        n519 = local read "DD"() -> (w1025:bool)
        n520 = local read "PS"() -> (w1024:bool)
        n521 = case shown="True" w1025 {
          frame False {
          }
          frame True {
            n522 = local read "DD"() -> (w1043:i32)
            n523 = Increment(x=w1043) -> (x+1=→"DD":i32)
          }
        }
        n524 = case shown="True" w1024 {
          frame False {
          }
          frame True {
            n525 = local read "PS"() -> (w1041:i32)
            n526 = Increment(x=w1041) -> (x+1=→"PS":i32)
          }
        }
        n527 = case shown="True" w1023 {
          frame False {
          }
          frame True {
            n528 = local read "ADC"() -> (w1039:i32)
            n529 = Increment(x=w1039) -> (x+1=→"ADC":i32)
          }
        }
        n530 = case shown="True" w1022 {
          frame False {
          }
          frame True {
            n531 = local read "STAB"() -> (w1037:i32)
            n532 = Increment(x=w1037) -> (x+1=→"STAB":i32)
          }
        }
        n533 = case shown="True" w1021 {
          frame False {
          }
          frame True {
            n534 = local read "-15"() -> (w1035:i32)
            n535 = Increment(x=w1035) -> (x+1=→"-15":i32)
          }
        }
        n536 = case shown="True" w1020 {
          frame False {
          }
          frame True {
            n537 = local read "1V"() -> (w1033:i32)
            n538 = Increment(x=w1033) -> (x+1=→"1V":i32)
          }
        }
        n539 = local read "RD"() -> (w1019:bool)
        n540 = local read "2V"() -> (w1017:bool)
        n541 = local read "PH"() -> (w1018:bool)
        n542 = case shown="True" w1018 {
          frame False {
          }
          frame True {
            n543 = local read "PH"() -> (w1029:i32)
            n544 = Increment(x=w1029) -> (x+1=→"PH":i32)
          }
        }
        n545 = case shown="True" w1019 {
          frame False {
          }
          frame True {
            n546 = local read "RD"() -> (w1031:i32)
            n547 = Increment(x=w1031) -> (x+1=→"RD":i32)
          }
        }
        n548 = case shown="True" w1017 {
          frame False {
          }
          frame True {
            n549 = local read "2V"() -> (w1027:i32)
            n550 = Increment(x=w1027) -> (x+1=→"2V":i32)
          }
        }
      }
      frame #3 {
        w1064 = i16 0 ("width (-)")
        w1067 = i16 3 ("width (-)")
        w1065 = "\t"
        # "Логирование данных"
        n551 = local read "STAB"() -> (w1062:i32)
        n552 = local read "ADC"() -> (w1063:i32)
        n553 = local read "-15"() -> (w1061:i32)
        n554 = local read "PH"() -> (w1058:i32)
        n555 = local read "DD"() -> (w1056:i32)
        n556 = local read "RD"() -> (w1059:i32)
        n557 = local read "1V"() -> (w1060:i32)
        n558 = local read "2V"() -> (w1057:i32)
        n559 = local read "PS"() -> (w1055:i32)
        n560 = Number To Fractional String(number=w1063, width (-)=w1064, precision (6)=w1064) -> (F-format string=w1052:string)  [unwired: 1 in]
        n561 = Number To Fractional String(number=w1062, width (-)=w1064, precision (6)=w1064) -> (F-format string=w1051:string)  [unwired: 1 in]
        n562 = Number To Fractional String(number=w1061, width (-)=w1064, precision (6)=w1064) -> (F-format string=w1050:string)  [unwired: 1 in]
        n563 = Number To Fractional String(number=w1060, width (-)=w1064, precision (6)=w1064) -> (F-format string=w1049:string)  [unwired: 1 in]
        n564 = Number To Fractional String(number=w1059, width (-)=w1064, precision (6)=w1064) -> (F-format string=w1048:string)  [unwired: 1 in]
        n565 = Number To Fractional String(number=w1058, width (-)=w1064, precision (6)=w1064) -> (F-format string=w1047:string)  [unwired: 1 in]
        n566 = Number To Fractional String(number=w1057, width (-)=w1064, precision (6)=w1064) -> (F-format string=w1046:string)  [unwired: 1 in]
        n567 = Number To Fractional String(number=w1056, width (-)=w1064, precision (6)=w1064) -> (F-format string=w1045:string)  [unwired: 1 in]
        n568 = Number To Fractional String(number=w1055, width (-)=w1064, precision (6)=w1064) -> (F-format string=w1044:string)  [unwired: 1 in]
        n569 = local read "PH_LOW_cur"() -> (w1071:dbl)
        n570 = local read "PS_LOW_cur"() -> (w1068:dbl)
        n571 = local read "STAB_cur"() -> (w1075:dbl)
        n572 = local read "ADC_cur"() -> (w1076:dbl)
        n573 = local read "DD_cur"() -> (w1069:dbl)
        n574 = local read "-15_cur"() -> (w1074:dbl)
        n575 = local read "RD_cur"() -> (w1072:dbl)
        n576 = local read "1V_cur"() -> (w1073:dbl)
        n577 = local read "2V_cur"() -> (w1070:dbl)
        n578 = Number To Fractional String(number=w1076, width (-)=w1067, precision (6)=w1067) -> (F-format string=w1085:string)  [unwired: 1 in]
        n579 = Number To Fractional String(number=w1075, width (-)=w1067, precision (6)=w1067) -> (F-format string=w1084:string)  [unwired: 1 in]
        n580 = Number To Fractional String(number=w1074, width (-)=w1067, precision (6)=w1067) -> (F-format string=w1083:string)  [unwired: 1 in]
        n581 = Number To Fractional String(number=w1073, width (-)=w1067, precision (6)=w1067) -> (F-format string=w1082:string)  [unwired: 1 in]
        n582 = Number To Fractional String(number=w1072, width (-)=w1067, precision (6)=w1067) -> (F-format string=w1081:string)  [unwired: 1 in]
        n583 = Number To Fractional String(number=w1071, width (-)=w1067, precision (6)=w1067) -> (F-format string=w1080:string)  [unwired: 1 in]
        n584 = Number To Fractional String(number=w1070, width (-)=w1067, precision (6)=w1067) -> (F-format string=w1079:string)  [unwired: 1 in]
        n585 = Number To Fractional String(number=w1069, width (-)=w1067, precision (6)=w1067) -> (F-format string=w1078:string)  [unwired: 1 in]
        n586 = Number To Fractional String(number=w1068, width (-)=w1067, precision (6)=w1067) -> (F-format string=w1077:string)  [unwired: 1 in]
        n587 = Get Date/Time In Seconds() -> (seconds since 1Jan1904=w1088:timestamp)
        n588 = Format Date/Time String(time format string (%c)="%d %H:%M:%S:%3u", seconds (now)=w1088) -> (date/time string=w1086:string)  [unwired: 1 in]
        n589 = Concatenate Strings(w1086, w1065, w1085, w1065, w1084, w1065, w1083, w1065, w1082, w1065, w1081, w1065, w1080, w1065, w1079, w1065, w1078, w1065, w1077, w1065, w1052, w1065, w1051, w1065, w1050, w1065, w1049, w1065, w1048, w1065, w1047, w1065, w1046, w1065, w1045, w1065, w1044, "\r\n") -> (w1087:string)
        n590 = Format Into String(initial string=w1054, w1087) -> ()  [unwired: 2 in, 2 out]
      }
      frame #4 {
        n591 = flat-sequence {
          frame #0 {
            n592 = local read "STAB"() -> (w1096:bool)
            n593 = local read "ADC"() -> (w1097:bool)
            n594 = local read "DD"() -> (w1099:bool)
            n595 = local read "-15"() -> (w1095:bool)
            n596 = local read "PS"() -> (w1098:bool)
            n597 = local read "1V"() -> (w1094:bool)
            n598 = local read "RD"() -> (w1093:bool)
            n599 = local read "PH"() -> (w1092:bool)
            n600 = local read "2V"() -> (w1091:bool)
            n601 = Compound Arithmetic op=OR(w1099, w1098, w1097, w1096, w1095, w1094, w1093, w1092, w1091) -> (w1090:bool)
            n602 = case shown="True" w1090 {
              selector: w1090 -> [_ w1101]
              frame False {
              }
              frame True {
                n603 = Not(x=w1101) -> (.not. x?=w1100:bool)
                n604 = local write "Питание"(w1100) -> ()
              }
            }
          }
          frame #1 {
            n605 = case shown="True" "Включаем автоматом?" {
              frame False {
              }
              frame True {
                n606 = flat-sequence {
                  frame #0 {
                    n607 = Wait (ms)(milliseconds to wait=u32 100) -> ()  [unwired: 1 out]
                  }
                  frame #1 {
                    n608 = local write "Питание"(TRUE ("Питание")) -> ()
                  }
                  frame #2 {
                    n609 = Wait (ms)(milliseconds to wait=u32 100) -> ()  [unwired: 1 out]
                  }
                }
              }
            }
          }
        }
        n610 = local read "Стоп"() -> (w1089:bool)
      }
    }
    n611 = Wait (ms)(milliseconds to wait=u32 1) -> ()  [unwired: 1 out]
  }
  n612 = while {
    tunnel: w1 -> [w1141]
    tunnel: [w1140] -> w3
    stop <- w1139 stop-if-true
    # "Общие настройки"
    n613 = local read "Питание"() -> (w1143:bool)
    n614 = case shown="\"MAX\"" "Частота?" {
      tunnel: ["CDS1_2" u8 6 ("CDS1_2")] -> w1130
      tunnel: ["CDS1_1" u8 3 ("CDS1_1")] -> w1129
      tunnel: ["CDS2_2" u8 7 ("CDS2_2")] -> w1128
      tunnel: ["CDS2_1" u8 1 ("CDS2_1")] -> w1127
      tunnel: ["ADC_2" u8 9 ("ADC_2")] -> w1126
      tunnel: ["ADC_1" u8 3 ("ADC_1")] -> w1125
      tunnel: ["RG_2" u8 8 ("RG_2")] -> w1124
      tunnel: ["HOR" u16 880 ("HOR")] -> w1123
      tunnel: ["LOW" u8 1 ("LOW")] -> w1122
      tunnel: ["HIGH" u8 9 ("HIGH")] -> w1121
      tunnel: ["RG_1" u8 2 ("RG_1")] -> w1113
      tunnel: ["PH21_2" u8 7 ("PH21_2")] -> w1112
      tunnel: ["PH21_1" u8 2 ("PH21_1")] -> w1111
      tunnel: ["PH11_2" u8 7 ("PH11_2")] -> w1110
      tunnel: ["PH11_1" u8 2 ("PH11_1")] -> w1109
      tunnel: ["10" u8 10 ("10")] -> w1108
      frame "MIN", Default {
      }
      frame "MAX" {
      }
    }
    n615 = And(x="Линейки", y=w1143) -> (x .and. y?=w1137:bool)
    n616 = local read "Стоп"() -> (w1138:bool)
    n617 = xnode "Read/Write Control"("FPGA VI Reference In"=w1141, "Остановка основного цикла"=w1138, "Линейки"=w1137, "Сколько строк?"="Сколько строк?", "Строка триггер"="Строка триггер", "2017"="2017", "PS1_2"="PS1_2", "PS1_1"="PS1_1", "PS2_1"="PS2_1", "PS2_2"="PS2_2", "PS3_1"="PS3_1", "PS3_2"="PS3_2", "PS4_1"="PS4_1", "PS4_2"="PS4_2", "CDS1_2"=w1130, "CDS1_1"=w1129, "CDS2_2"=w1128, "CDS2_1"=w1127, "ADC_2"=w1126, "ADC_1"=w1125, "RG_2"=w1124, "RG_1"=w1113, "PH21_2"=w1112, "PH21_1"=w1111, "PH11_2"=w1110, "PH11_1"=w1109, "HOR"=w1123, "10"=w1108, "LOW"=w1122, "HIGH"=w1121, "Направление бит"=FALSE, "Между кадрами"="Между кадрами, мс") -> ("FPGA VI Reference Out"=w1140:refnum<k20>)  [unwired: 1 in, 1 out]
    n618 = Wait (ms)(milliseconds to wait=u32 1) -> ()  [unwired: 1 out]
    n619 = local read "Стоп"() -> (w1139:bool)
  }
  n620 = call <instrlib>:"niDCPower Close.vi"("instrument handle"=w6) -> ()  [unwired: 10 in, 1 out]
  n621 = xnode "Close FPGA VI Reference"("FPGA VI Reference In"=w3) -> ()  [unwired: 1 in, 1 out]
  n622 = call <instrlib>:"niDCPower Close.vi"("instrument handle"=w7) -> ()  [unwired: 10 in, 1 out]
  n623 = call <instrlib>:"niDCPower Close.vi"("instrument handle"=w8) -> ()  [unwired: 10 in, 1 out]
